vi "信号光谱7.vi"() -> ()   [LabVIEW 2018]
uses:
  <vilib>/Utility/NIReport.llb/Report Type.ctl
  <vilib>/Utility/file.llb/Write Delimited Spreadsheet (DBL).vi
  <vilib>/Instr/_visa.llb/VISA Configure Serial Port (Instr).vi
  <vilib>/addons/_office/excel.llb/Excel Get Data ([str]).vi
  <vilib>/Utility/NIReport.llb/NI_report.lvclass
  <vilib>/Analysis/NI_AALBase.lvlib
  <vilib>/ptbypt/NI_PtbyPt.lvlib
  <vilib>/Utility/NIReport.llb/NI_ReportGenerationCore.lvlib
  <vilib>/addons/_office/NI_ReportGenerationToolkit.lvlib
  <vilib>/Utility/NIReport.llb/Excel/NI_Excel.lvclass
panel:
  in  "终止测量":bool
  in  "测量次数":i32=10
  out "best fit":cluster{"Y":dbl[], "Y":dbl[]}[](graph)
  in  "拟合终点":i32=700
  in  "拟合起点":i32=350
  out "angle":dbl
  out "图片地址":string
  in  "开光时间/ms":u32=500
  out "最终存储路径 2":path
  out "照明光error out":errorcluster
  in  "照明光":bool
  in  "stop bits (10: 1 bit)":u16(ring)=10 items=["1.0"=10, "1.5"=15, "2.0"=20]
  in  "parity (0:none)":enum16{"None", "Odd", "Even", "Mark", "Space"}(ring)
  in  "data bits (8)":u16=8 min=5 max=8 step=1
  in  "baud rate":u32=9600 caption="baud rate (115200)" min=9600 max=115200
  in  "照明光VISA":refnum<visa-resource-name>="COM7"
  out "正在测量":bool
  in  "滤波阈值":dbl=1500.0 format="%#_13g"
  out "范围内？":bool[](array[boolean])
  out "w":dbl
  out "xc":dbl
  out "拟合参数":dbl[](array[numeric])
  out "最终存储路径":path
  in  "停止程序":bool
  in  "上升下降沿/s":dbl format="%.2p"
  in  "延时/s":dbl format="%.2p"
  in  "占空比/%":dbl=3.0 format="%.2p"
  in  "高电平/V":dbl=4.0 format="%.2p"
  in  "频率/Hz":dbl=6000.0 format="%.3p"
  in  "低电平/V":dbl min=0.0 max=5.0 format="%.2p"
  out "configure error out":errorcluster
  in  "设置参数":bool
  out "output control error  4":errorcluster
  in  "低电平持续输出":bool
  in  "Output 1":bool
  out "output control error  5":errorcluster
  in  "测量高电平/V":dbl=4.0
  out "output control error":errorcluster
  in  "开始测量":bool
  in  "上升下降沿":i32(ring)=1 items=["上升沿", "下降沿"]
  in  "channel输出口":i32(ring) items=["Channel 1", "Channel 2"]
  in  "输出信号波形":u16(ring) items=["Pulse"]
  out "output control error":errorcluster
  out "Output":bool
  in  "VISA 信号发生器":refnum<visa-resource-name>="USB0::0x1AB1::0x0641::DG4E192200870::INSTR"
  out "Spectrum":cluster{"Y":dbl[], "Y":dbl[]}[](graph)
  out "波长范围":dbl[](array[numeric])
  in  "选项卡控件":enum32{"IHR 550", "CCD"}(tab)
  in  "Move To\nTarget Positions":bool
  out "Current UniqueID":string="Mono4"
  in  "Mono ID":string(combo)="Mono1"
  in  "Connect":bool
  out "Initialized JY":bool=TRUE
  in  "Force\nInitialization":bool
  in  "Target Grating":string(combo)="2"
  out "Current Description":string="1" caption="Description"
  out "Grating Index":i32=1
  out "Current Grating":dbl=1200.0
  out "Units":string="nm"
  out "Current WL":dbl=897.9988
  out "Exit Mirror\nPosition":i32(ring)=2 items=["EntranceMirror", "ExitMirror", "Front", "Side"]
  out "Entrance Mirror\nPosition":i32(ring)=2 items=["EntranceMirror", "ExitMirror", "Front", "Side"]
  out "Units 2":string="mm"
  out "Front Entrance":dbl
  in  "Target WL":dbl=2670.0
  in  "Exit Mirror":u16(ring)=3 caption="Target Position Exit Mirror" items=["Front"=2, "Side"=3]
  in  "Entrance Mirror":u16(ring)=2 caption="Target Position\nEntrance Mirror" items=["Front"=2, "Side"=3]
  in  "Target\nFront Entrance":dbl=1.0
  in  "Commande tab":T1(tab)
  in  "Area Number to Display":i32
  in  "Reformat":bool
  in  "GAIN":u16(ring)=2 caption="Device Name" items=["High Light", "Best Dynamic Range", "High Sensitivity"]
  in  "ADC":u16(ring) caption="Device Name" items=["20 kHz       ", " 1 MHz       ", " 1 MHz Ultra "]
  in  "Number of Areas :":u16=1 min=1 step=1
  in  "Integration time (ms) :":i16=10000
  out "Uniques ID":u16(ring) items=["CCD1", "CCD2"]
  in  "Device Name":u16(ring) items=["Synapse CCD (Lateral)", "Synapse_IGA (Axial)"]
  in  "Signal type :":enum16{"TTL Rising Edge", "TTL Falling Edge"}(ring)=enum."TTL Falling Edge"
  in  "Trigger Type :":u16(ring) items=["On Start"=1, "Per Acquisition"=2]
  in  "trigSigTypeString":string
  in  "trigEventString":string
  in  "Enable InputTriggers :":bool
  in  "Number of Cleans":i32=1
  in  "MultiAcqShutterMode":i32(ring)=3 items=["Open For All Spectra"=1, "Open for Each Spectrum"=3]
  in  "Accumulations:":u16=10 min=1 step=1
  in  "Multi Accumulation mode:":bool
  out "Y Pixels:":i32=256
  out "DataSize":i32=1024
  out "X Pixels:":i32=1024
  out "Firmware\nVersion":string="V1.20 CCD_4000"
  out "initialized ?":bool=TRUE
  in  "Continuous":bool
  in  "CCD Busy":bool
  out "indicator":string="Ready !"
  in  "initialize":bool
  in  "ShutterOpen":bool=TRUE caption="Shutter enable"
  in  "Acquire":bool
  in  "Temperature":bool
  in  "Setup":bool
  out "Acq Time(ms)":u32=3401
  in  "Save Backlight":bool
  in  "cut backlight":bool
  out "backlight":bool=TRUE
  in  "是否拟合":bool
  in  "是否保存":bool
  in  "Close":bool=TRUE
  out "JYCCDLib.IJYCCDReqd":refnum<k7>
  out "areas :":i32[][](array[numeric])=[[1], [1], [1], [1024], [256], [1], [256]]
  in  "Constante de condition\n(Voir l'aide contextuelle)":bool
  out "temp graph":dbl(graph)=-134.538067
  out "ADC Number":i32[](array[numeric])=[0, 1, 2, 3, 4]
  out "Gain Number":i32[](array[numeric])=[10, 11, 12, 13, 8, 2]
  out "trigAddress":i32
  out "Data":i32[][](graph)
  out "error out":errorcluster
  out "Gratings":dbl[](array[numeric])=[1200.0, 300.0]
  out "Backlight":i32[][](graph)
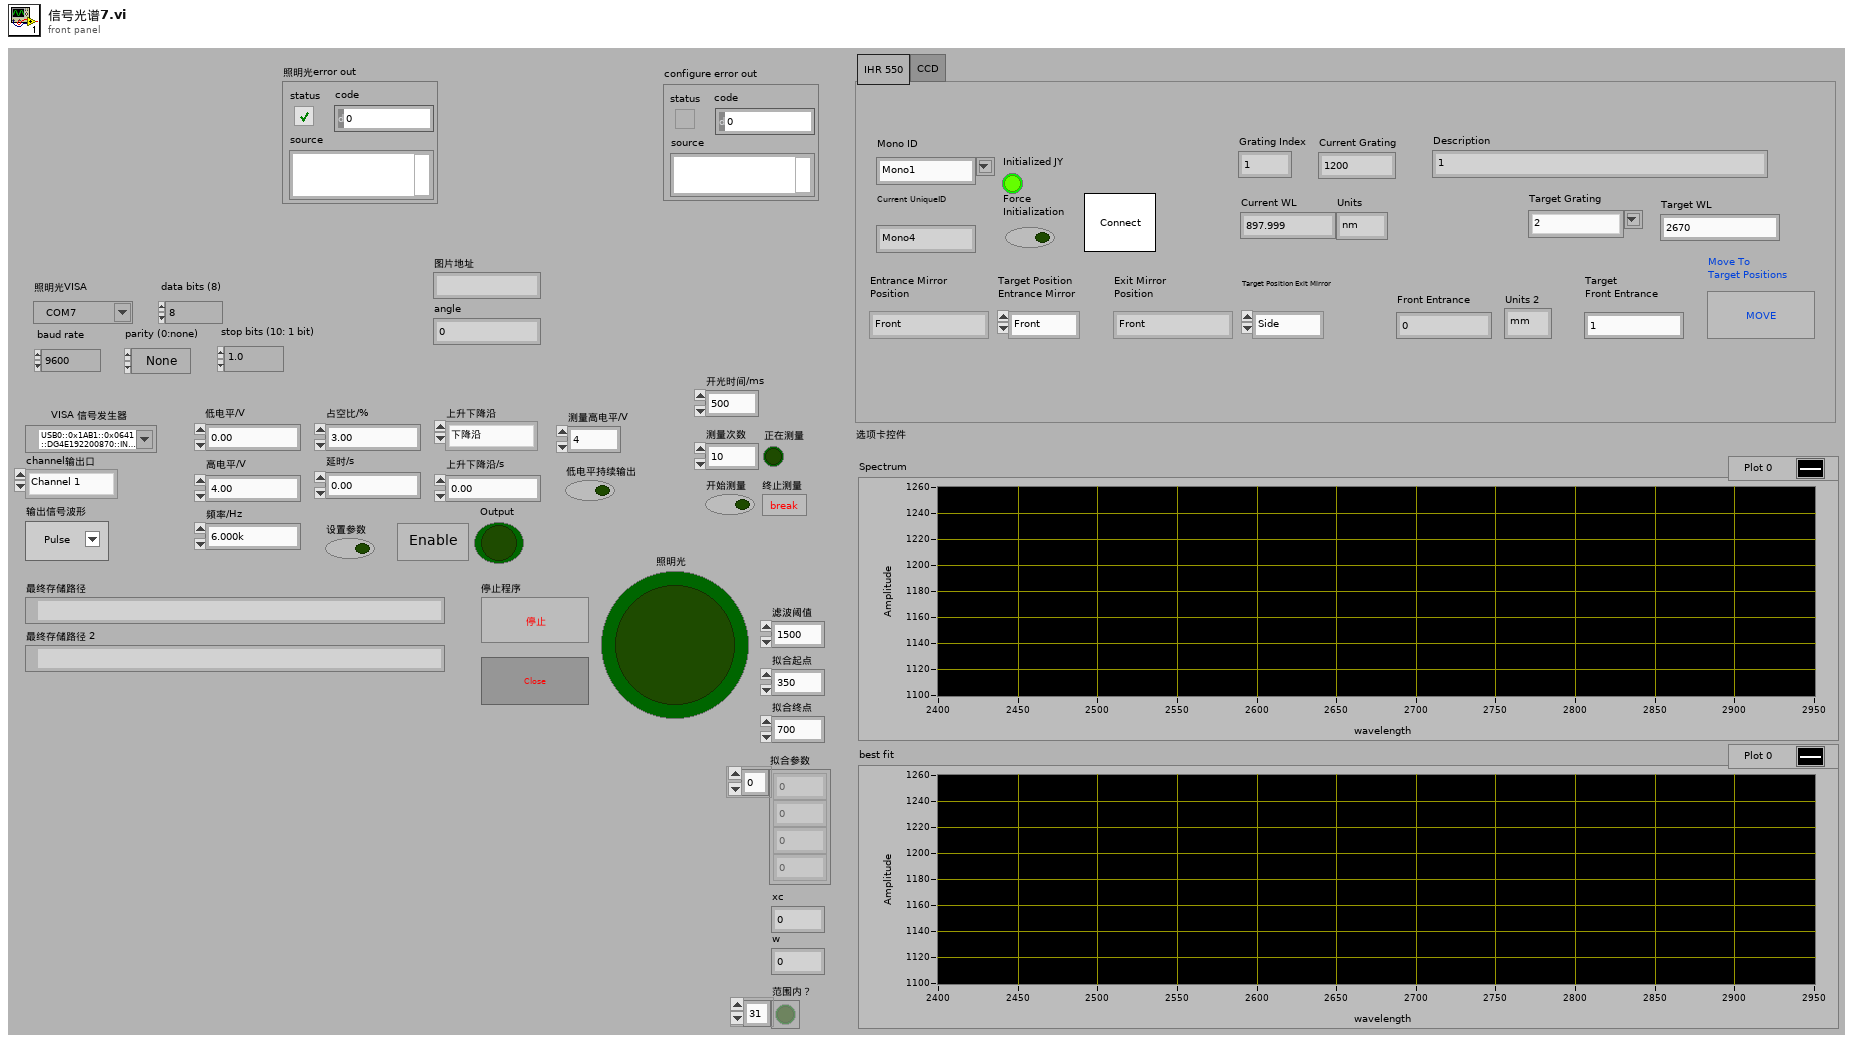
[diagram p1: front panel]
types:
  T1 = enum32{"Settings", "Trigger In", "Multi-Accu.", "Infos"}
  T2 = enum8{"Enabled", "Disabled", "Disabled and Grayed Out"}
  T3 = enum16{"maximized", "minimized", "normal", "no change"}
  T4 = typedef "NI_ReportGenerationCore.lvlib/Report Type.ctl" = enum16{"HTML", "Word", "Excel"}
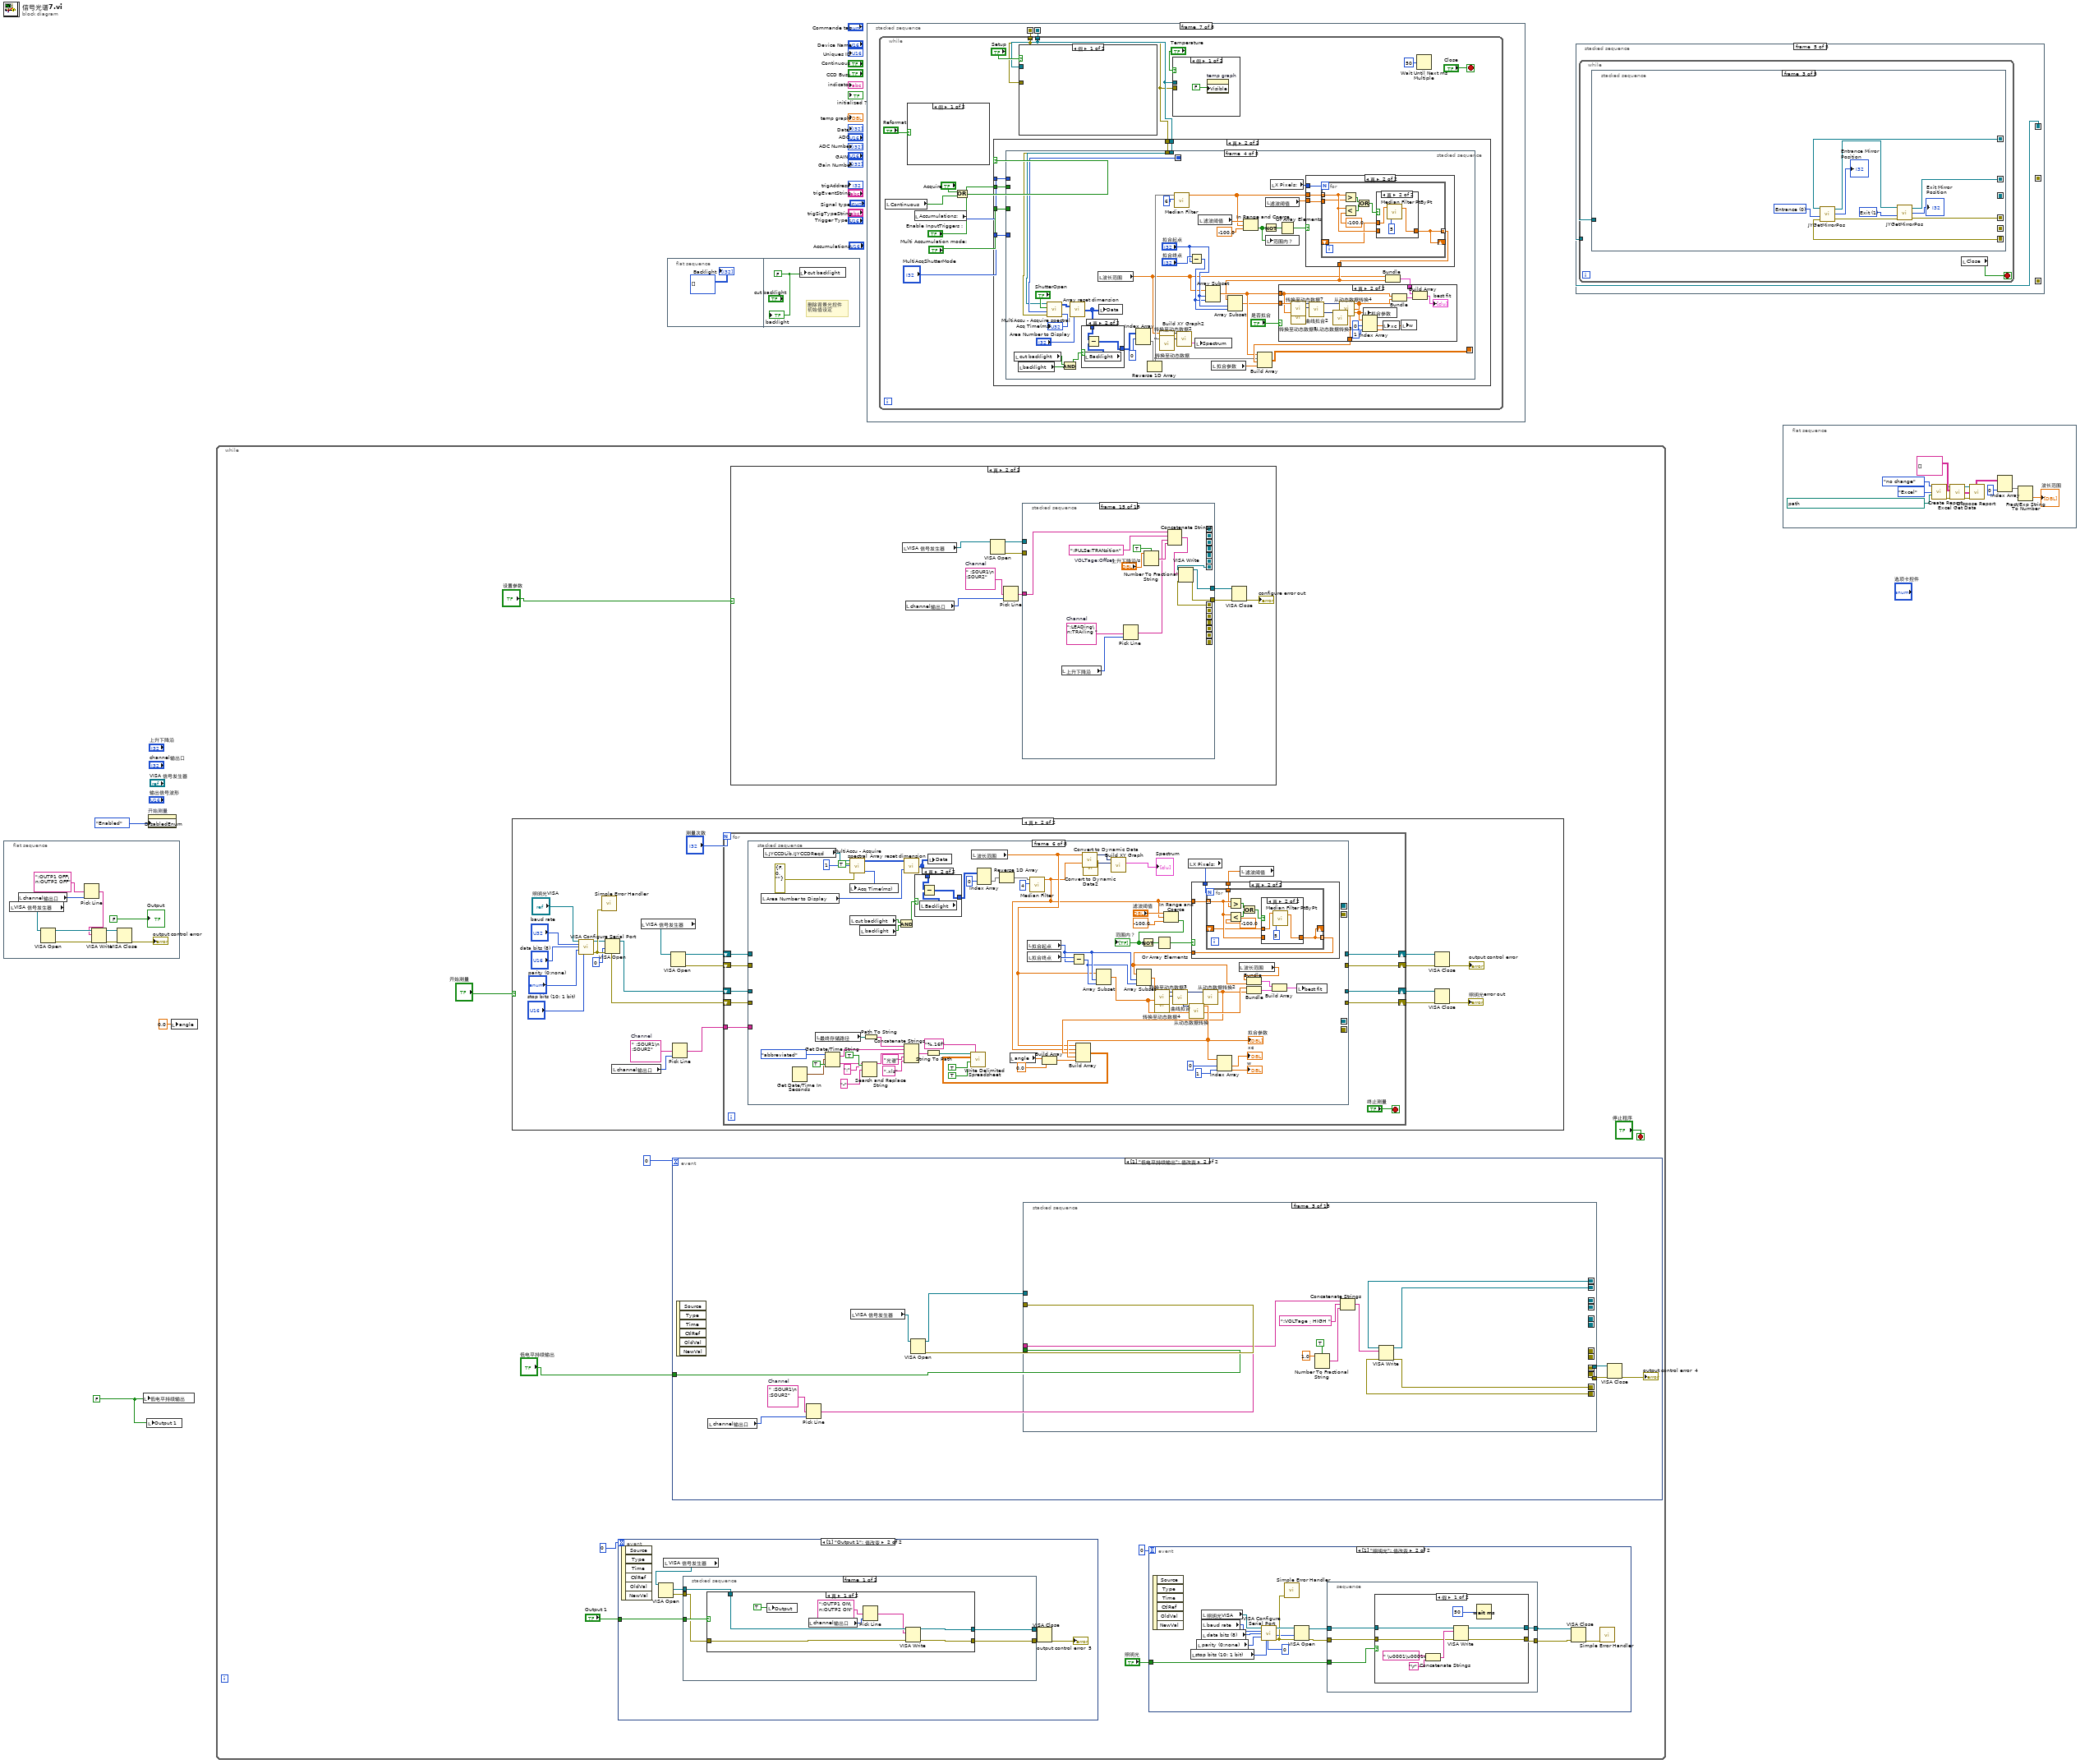
[diagram p0: block diagram]
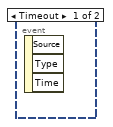
[diagram p2: hidden frame]
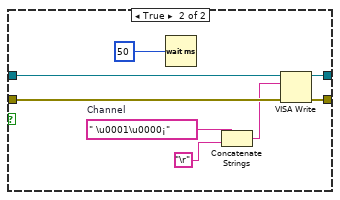
[diagram p3: hidden frame]
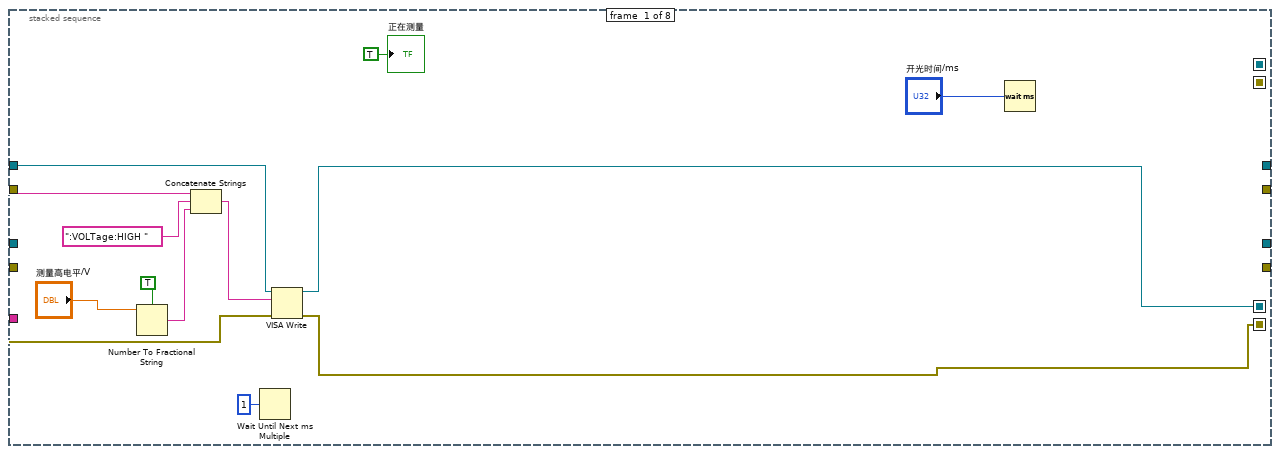
[diagram p5: hidden frame]
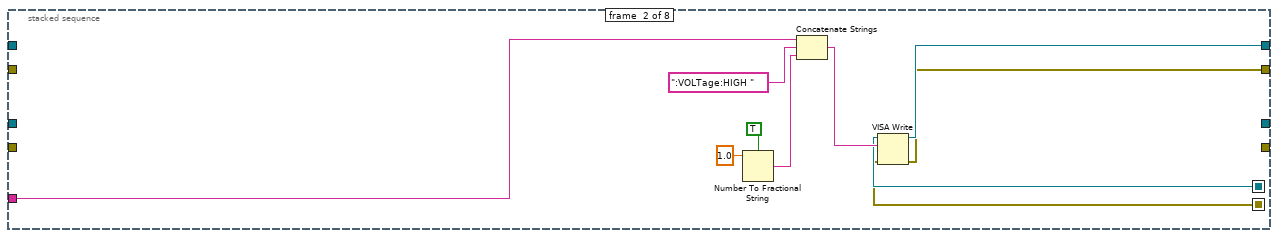
[diagram p6: hidden frame]
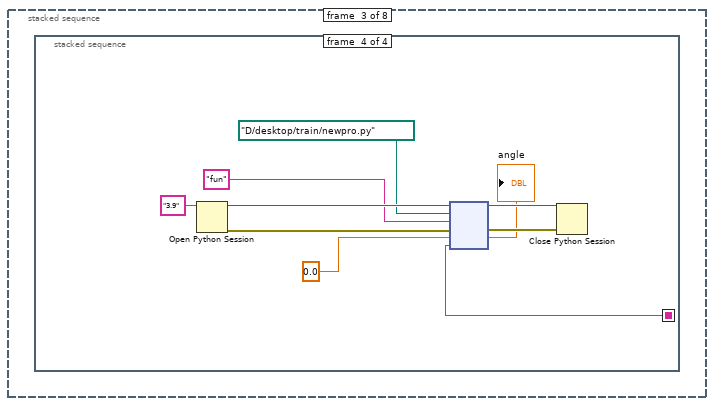
[diagram p7: hidden frame]
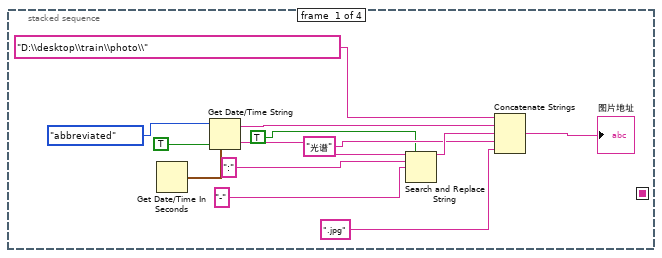
[diagram p8: hidden frame]
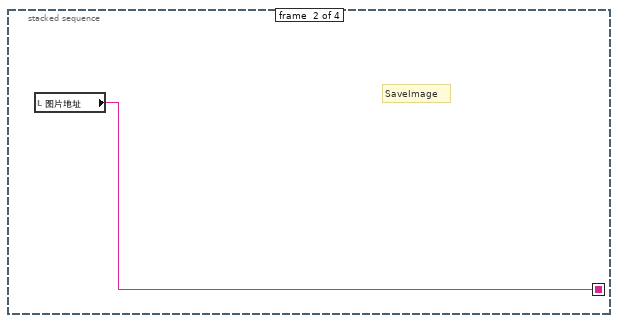
[diagram p9: hidden frame]
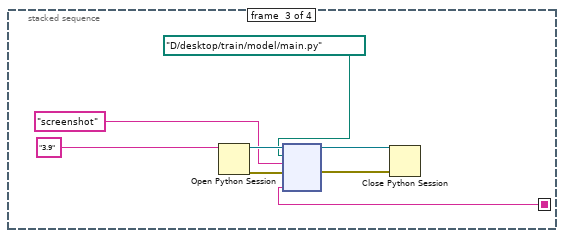
[diagram p10: hidden frame]
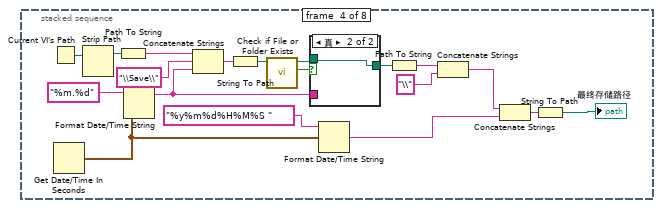
[diagram p11: hidden frame]
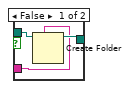
[diagram p12: hidden frame]
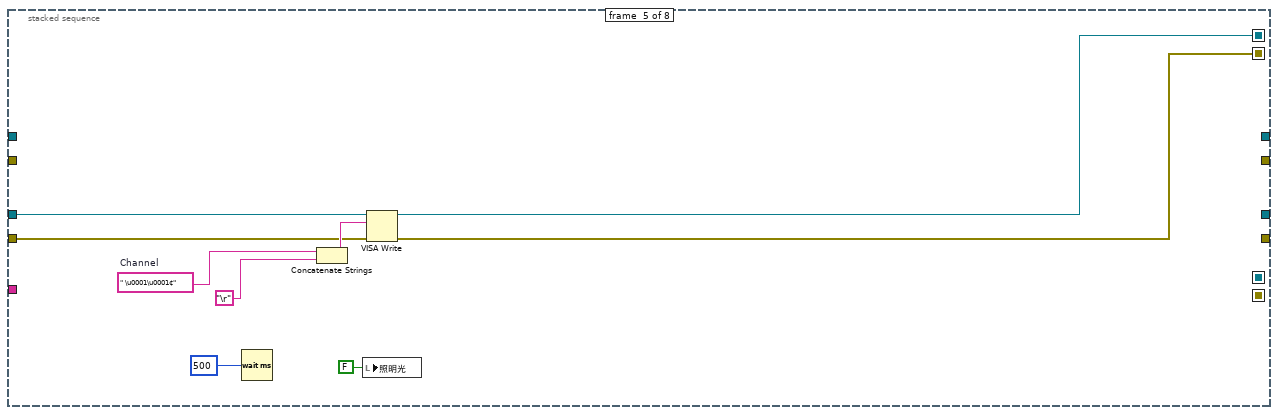
[diagram p13: hidden frame]
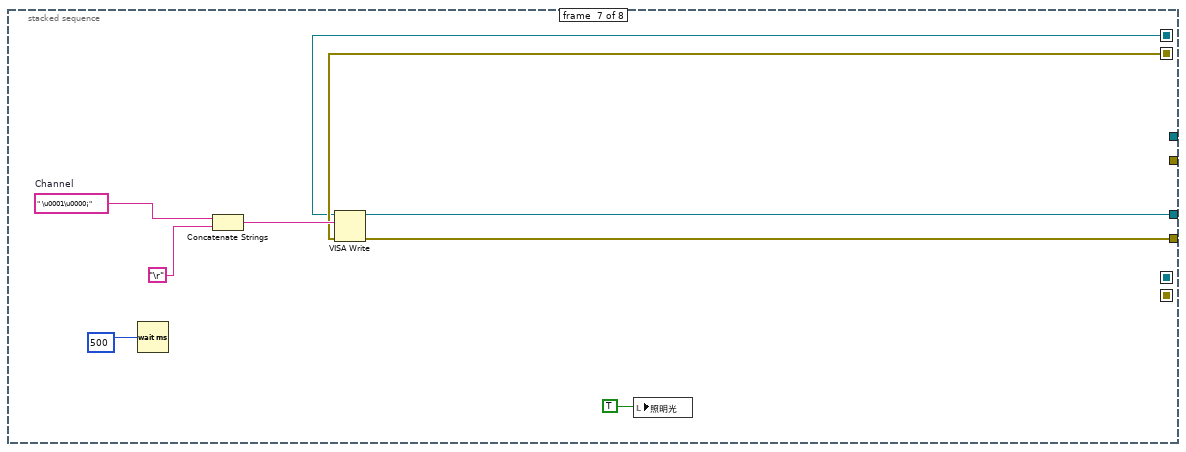
[diagram p17: hidden frame]
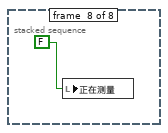
[diagram p18: hidden frame]
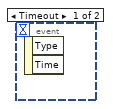
[diagram p19: hidden frame]
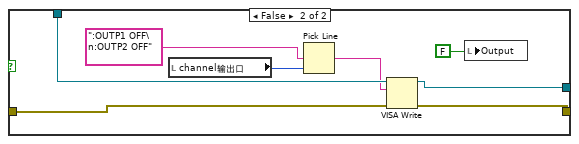
[diagram p20: hidden frame]
diagram:
  w2 = FALSE
  n1 = flat-sequence {
    frame #0 {
      n2 = local read "VISA 信号发生器"() -> (w7:refnum<visa-resource-name>)
      n3 = local read "channel输出口"() -> (w5:i32)
      n4 = VISA Open(VISA resource name=w7) -> (VISA resource name=w13:refnum<visa-resource-name>, error out=w12:errorcluster)  [unwired: 4 in]
      n5 = Pick Line(multi-line string=":OUTP1 OFF\n:OUTP2 OFF" ("write buffer"), line index=w5) -> (output string=w4:string)  [unwired: 1 in]
      n6 = VISA Write(VISA resource name=w13, write buffer=w4, error in (no error)=w12) -> (VISA resource name out=w10:refnum<visa-resource-name>, error out=w9:errorcluster)  [unwired: 1 out]
      n7 = VISA Close(VISA resource name=w10, error in (no error)=w9) -> (error out=→"output control error":errorcluster)
      "Output" <- FALSE ("布尔")
    }
  }
  n8 = local write "低电平持续输出"(w2) -> ()
  n9 = local write "Output 1"(w2) -> ()
  n10 = property on="开始测量" class="Bool"("DisabledEnum"=T2."Enabled" ("禁用")) -> ()  [unwired: 2 in, 2 out]
  n11 = local write "angle"(0.0 ("angle")) -> ()
  n12 = while {
    stop <- "停止程序" stop-if-true
    n13 = case shown="真" "开始测量" {
      frame False {
      }
      frame True {
        w74 = " :SOUR1\n :SOUR2"  # Channel
        n14 = call-poly "VISA Configure Serial Port"("VISA resource name"="照明光VISA", "baud rate (9600)"="baud rate", "data bits (8)"="data bits (8)", "parity (0:none)"="parity (0:none)", "stop bits (10: 1 bit)"="stop bits (10: 1 bit)") -> ("VISA resource name out"=w69:refnum<visa-resource-name>, "error out"=w70:errorcluster)  [unwired: 9 in]
        n15 = call <vilib>:"Simple Error Handler.vi"("error in (no error)"=w70) -> ()  [unwired: 4 in, 5 out]
        n16 = VISA Open(access mode=0, error in (no error)=w70, VISA resource name=w69) -> (VISA resource name=w62:refnum<visa-resource-name>, error out=w61:errorcluster)  [unwired: 2 in]
        n17 = local read "channel输出口"() -> (w75:i32)
        n18 = local read "VISA 信号发生器"() -> (w80:refnum<visa-resource-name>)
        n19 = VISA Open(VISA resource name=w80) -> (VISA resource name=w79:refnum<visa-resource-name>, error out=w78:errorcluster)  [unwired: 4 in]
        n20 = Pick Line(multi-line string=w74, line index=w75) -> (output string=w73:string)  [unwired: 1 in]
        n21 = for {
          N: "测量次数" -> [_]
          tunnel: w73 -> [w88]
          shift-right: [w84] -> w72
          shift-left: w79 -> [w90]
          shift-right: [w83] -> w71
          shift-left: w78 -> [w89]
          shift-right: [w82] -> w77
          shift-left: w62 -> [w87]
          shift-right: [w81] -> w76
          shift-left: w61 -> [w86]
          stop <- "终止测量" stop-if-true
          n22 = stacked-sequence {
            seq-local: [w95 _ _ _ _ _ _ _] -> [_ w106 _ _ _ _ _ _]
            seq-local: [w94 _ _ _ _ _ _ _] -> [_ w105 _ _ _ _ _ _]
            seq-local: [_ _ _ _ w171 _ _ _] -> [_ _ _ _ _ _ w271 _]
            seq-local: [_ _ _ _ w170 _ _ _] -> [_ _ _ _ _ _ w274 _]
            tunnel: w90 -> [w98 _ _ _ _ _ _ _]
            tunnel: w89 -> [w97 _ _ _ _ _ _ _]
            tunnel: [_ w108 _ _ _ _ _ _] -> w84
            tunnel: [_ w107 _ _ _ _ _ _] -> w83
            tunnel: w88 -> [w99 w104 _ _ _ _ _ _]
            tunnel: w87 -> [_ _ _ _ w174 _ _ _]
            tunnel: w86 -> [_ _ _ _ w173 _ _ _]
            tunnel: [_ _ _ _ _ _ w273 _] -> w82
            tunnel: [_ _ _ _ _ _ w272 _] -> w81
            frame #0 {
              n23 = Number To Fractional String(use system decimal point (T)=TRUE ("使用系统小数点(T)"), number="测量高电平/V") -> (F-format string=w101:string)  [unwired: 2 in]
              n24 = Concatenate Strings ("连接字符串")(w99, ":VOLTage:HIGH ", w101) -> (w100:string)
              n25 = Wait Until Next ms Multiple(millisecond multiple=u32 1 ("毫秒倍数")) -> ()  [unwired: 1 out]
              n26 = VISA Write(VISA resource name=w98, write buffer=w100, error in (no error)=w97) -> (VISA resource name out=w95:refnum<visa-resource-name>, error out=w94:errorcluster)  [unwired: 1 out]
              n27 = Wait (ms)(milliseconds to wait="开光时间/ms") -> ()  [unwired: 1 out]
              "正在测量" <- TRUE
            }
            frame #1 {
              n28 = Number To Fractional String(use system decimal point (T)=TRUE ("使用系统小数点(T)"), number=1.0 ("数字")) -> (F-format string=w111:string)  [unwired: 2 in]
              n29 = Concatenate Strings ("连接字符串")(w104, ":VOLTage:HIGH ", w111) -> (w110:string)
              n30 = VISA Write(VISA resource name=w106, write buffer=w110, error in (no error)=w105) -> (VISA resource name out=w108:refnum<visa-resource-name>, error out=w107:errorcluster)  [unwired: 1 out]
            }
            frame #2 {
              n31 = stacked-sequence {
                seq-local: [_ w127 _ _] -> [_ _ w128 w136]
                frame #0 {
                  n32 = Get Date/Time In Seconds() -> (seconds since 1Jan1904=w123:timestamp)
                  n33 = Get Date/Time String(date format (0)=enum16{"short", "long", "abbreviated"}."abbreviated" ("日期格式(0)"), seconds (now)=w123, want seconds? (F)=TRUE ("需要秒？(F)")) -> (date string=w126:string, time string=w124:string)
                  n34 = Search and Replace String(replace all?=TRUE ("替换全部？(F)"), input string=w124, search string=":" ("搜索字符串"), replace string="-" ("替换字符串(\"\")")) -> (result string=w125:string)  [unwired: 4 in, 3 out]
                  n35 = Concatenate Strings("D:\\desktop\\train\\photo\\", w126, w125, "光谱" ("字符串"), ".jpg" ("字符串")) -> (→"图片地址":string)
                }
                frame #1 {
                  # "SaveImage"
                  n36 = local read "图片地址"() -> (w127:string)
                }
                frame #2 {
                  n37 = Open Python Session(python version="3.9" ("Python version")) -> (session out=w135:refnum<k35>, error out=w133:errorcluster)  [unwired: 2 in]
                  n38 = node(w135, path "D:/desktop/train/model/main.py" ("module path"), "screenshot" ("function name"), w133, w128) -> (w134:refnum<k35>, w132:errorcluster)  [unwired: 3 in, 2 out]
                  n39 = Close Python Session(session in=w134, error in=w132) -> ()  [unwired: 1 out]
                }
                frame #3 {
                  n40 = Open Python Session(python version="3.9" ("Python version")) -> (session out=w144:refnum<k35>, error out=w142:errorcluster)  [unwired: 2 in]
                  n41 = node(w144, path "D:/desktop/train/newpro.py" ("module path"), "fun" ("function name"), w142, 0.0, w136) -> (w143:refnum<k35>, w141:errorcluster, →"angle":dbl)  [unwired: 1 in, 2 out]
                  n42 = Close Python Session(session in=w143, error in=w141) -> ()  [unwired: 1 out]
                }
              }
            }
            frame #3 {
              n43 = Current VI's Path() -> (path=w151:path)
              n44 = Get Date/Time In Seconds() -> (seconds since 1Jan1904=w153:timestamp)
              n45 = Strip Path(path=w151) -> (stripped path=w152:path)  [unwired: 1 out]
              n46 = Path To String(path=w152) -> (string=w154:string)
              n47 = Format Date/Time String(time format string (%c)="%m.%d" ("时间格式字符串(%c)"), seconds (now)=w153) -> (date/time string=w160:string)  [unwired: 1 in]
              n48 = Concatenate Strings(w154, "\\Save\\" ("字符串"), w160) -> (w155:string)
              n49 = String To Path(string=w155) -> (path=w156:path)
              n50 = call <vilib>:"Check if File or Folder Exists.vi"("path"=w156) -> ("file or folder exists?"=w157:bool, "dup path"=w159:path)  [unwired: 8 in, 1 out]
              n51 = case shown="真" w157 {
                tunnel: [w167 w168] -> w158
                tunnel: w159 -> [w166 w168]
                tunnel: w160 -> [w165 _]
                frame False {
                  n52 = Create Folder(prompt (Create Folder)=w165, path (use dialog)=w166) -> (created path=w167:path)  [unwired: 1 in, 2 out]
                }
                frame True {
                }
              }
              n53 = Format Date/Time String(time format string (%c)="%y%m%d%H%M%S " ("时间格式字符串(%c)"), seconds (now)=w153) -> (date/time string=w163:string)  [unwired: 1 in]
              n54 = Path To String(path=w158) -> (string=w161:string)
              n55 = Concatenate Strings(w161, "\\" ("字符串")) -> (w162:string)
              n56 = Concatenate Strings(w162, w163) -> (w150:string)
              n57 = String To Path(string=w150) -> (path=→"最终存储路径":path)
            }
            frame #4 {
              w169 = " \u0001\u0001¢"  # Channel
              n58 = Wait (ms)(milliseconds to wait=500) -> ()  [unwired: 1 out]
              n59 = Concatenate Strings(w169, "\r") -> (w175:string)
              n60 = local write "照明光"(FALSE ("照明光")) -> ()
              n61 = VISA Write(VISA resource name=w174, write buffer=w175, error in (no error)=w173) -> (VISA resource name out=w171:refnum<visa-resource-name>, error out=w170:errorcluster)  [unwired: 1 out]
            }
            frame #5 {
              n62 = local read "Area Number to Display"() -> (w221:i32)
              n63 = local read "JYCCDLib.IJYCCDReqd"() -> (w217:refnum<k7>)
              n64 = Get Date/Time In Seconds() -> (seconds since 1Jan1904=w230:timestamp)
              n65 = local read "最终存储路径"() -> (w244:path)
              n66 = Get Date/Time String(date format (0)=enum16{"short", "long", "abbreviated"}."abbreviated" ("日期格式(0)"), seconds (now)=w230, want seconds? (F)=TRUE ("需要秒？(F)")) -> (date string=w238:string, time string=w233:string)
              n67 = call "MultiAccu - Acquire spectral.vi"("error in"=errorcluster {"status"=FALSE, "code"=0, "source"=""}, "Accumulations:"=u16 1, "ShutterOpen"=TRUE, "JYCCDLib.IJYCCDReqd"=w217) -> ("Acq Time(ms)"=w223:u32, "Array Out"=w222:i32[][][])  [unwired: 1 out]
              n68 = local write "Acq Time(ms)"(w223) -> ()
              n69 = local read "cut backlight"() -> (w203:bool)
              n70 = local read "backlight"() -> (w201:bool)
              n71 = Search and Replace String(replace all?=TRUE ("替换全部？(F)"), input string=w233, search string=":" ("搜索字符串"), replace string="-" ("替换字符串(\"\")")) -> (result string=w237:string)  [unwired: 4 in, 3 out]
              n72 = Path To String(path=w244) -> (string=w227:string)
              n73 = And(x=w203, y=w201) -> (x .and. y?=w202:bool)
              n74 = call "Array reset dimension.vi"("Area Number"=w221, "Array In"=w222) -> ("Array Out"=w205:i32[][])
              n75 = Concatenate Strings(w227, w238, w237, "光谱" ("字符串"), ".xls" ("字符串")) -> (w242:string)
              n76 = case shown="真" w202 {
                tunnel: [w265 w267] -> w204
                tunnel: w205 -> [w265 w266]
                frame False {
                }
                frame True {
                  n77 = local read "Backlight"() -> (w268:i32[][])
                  n78 = Subtract(x=w266, y=w268) -> (x-y=w267:i32[][])
                }
              }
              n79 = String To Path(string=w242) -> (path=w243:path)
              n80 = local write "Data"(w205) -> ()
              n81 = local read "波长范围"() -> (w182:dbl[])
              n82 = Index Array(array=w204, index (row)=0 ("索引 (行)")) -> (element=w245:i32[])  [unwired: 1 in]
              n83 = Reverse 1D Array(array=w245) -> (reversed array=w246:i32[])
              n84 = local read "angle"() -> (w180:dbl)
              n85 = local read "拟合起点"() -> (w191:i32)
              n86 = local read "拟合终点"() -> (w193:i32)
              n87 = call <vilib>:"Median Filter.vi"("left rank"=4, "X"=w246) -> ("Filtered X"=w181:dbl[])  [unwired: 8 in, 1 out]
              n88 = Build Array(w180, 0.0 ("元素")) -> (w178:dbl[])
              n89 = Subtract(x=w193, y=w191) -> (x-y=w190:i32)
              n90 = call "Convert to Dynamic Data"("Array"=w182) -> ("Dynamic Data Type"=w214:dynamicdata)  [unwired: 3 in]
              n91 = call "Convert to Dynamic Data2"("Array"=w181) -> ("Dynamic Data Type"=w213:dynamicdata)  [unwired: 3 in]
              n92 = Array Subset(array=w182, index=w191, length=w190) -> (w188:dbl[])
              n93 = call "Build XY Graph"("Y Input"=w213, "X Input"=w214) -> ("XY Graph"=→"Spectrum":cluster{"Y":dbl[], "Y":dbl[]}[])  [unwired: 8 in, 1 out]
              n94 = call "转换至动态数据4"("Array"=w188) -> ("Dynamic Data Type"=w211:dynamicdata)  [unwired: 3 in]
              n95 = In Range and Coerce(upper limit="滤波阈值", x=w181, lower limit=-100.0) -> (In Range?=w196:bool[])  [unwired: 1 out]
              "范围内？" <- w196
              n96 = Not(x=w196) -> (.not. x?=w195:bool[])
              n97 = Or Array Elements(Boolean array=w195) -> (logical OR=w198:bool)
              n98 = local read "X Pixels:"() -> (w197:i32)
              n99 = local read "波长范围"() -> (w183:dbl[])
              n100 = local read "滤波阈值"() -> (w194:dbl)
              n101 = case shown="真" w198 {
                tunnel: w197 -> [_ w252]
                tunnel: w181 -> [w248 w251]
                tunnel: [w248 w250] -> w189
                tunnel: w194 -> [_ w249]
                frame False {
                }
                frame True {
                  n102 = for {
                    N: w252 -> [_]
                    tunnel: w251 -> [w256] mode=indexing
                    tunnel: [w255] -> w250 mode=indexing
                    shift-right: [w255] -> _
                    shift-left: _ -> [w254]
                    tunnel: w249 -> [w253]
                    n103 = Greater?(x=w256, y=w253) -> (0:w258:bool)
                    n104 = Less?(x=w256, y=-100.0) -> (x < y?=w259:bool)
                    n105 = Or(x=w258, y=w259) -> (x .or. y?=w257:bool)
                    n106 = case shown="真" w257 {
                      tunnel: w256 -> [w261 _]
                      tunnel: [w261 w263] -> w255
                      tunnel: w254 -> [_ w264]
                      frame False {
                      }
                      frame True {
                        n107 = call <vilib>:"Median Filter PtByPt.vi"("rank"=5, "x"=w264) -> ("Filtered x"=w263:dbl)  [unwired: 2 in, 1 out]
                      }
                    }
                  }
                }
              }
              n108 = Array Subset(array=w189, index=w191, length=w190) -> (w192:dbl[])
              n109 = call "转换至动态数据3"("Array"=w192) -> ("Dynamic Data Type"=w212:dynamicdata)  [unwired: 3 in]
              n110 = call "曲线拟合"("Locations"=w211, "Signals"=w212) -> ("best fit"=w216:dynamicdata, "non-linear coefficients"=w215:dynamicdata)  [unwired: 5 in, 3 out]
              n111 = call "从动态数据转换"("Dynamic Data Type"=w215) -> ("Array"=w208:dbl[])  [unwired: 3 in]
              "拟合参数" <- w208
              n112 = call "从动态数据转换2"("Dynamic Data Type"=w216) -> ("Array"=w187:dbl[])  [unwired: 3 in]
              n113 = Build Array(w182, w181, w187, w208, w178) -> (w247:dbl[][])
              n114 = call-poly <vilib>:"Write Delimited Spreadsheet.vi"("file path (dialog if empty)"=w243, "format (%.3f)"="%.16f", "2D data"=w247, "append to file? (new file:F)"=TRUE ("append to file? (F)"), "transpose? (no:F)"=TRUE ("transpose? (F)")) -> ()  [unwired: 9 in, 2 out]
              n115 = Index Array(array=w208, index #1=0 ("索引"), index #2=1 ("索引")) -> (element #1=→"xc":dbl, element #2=→"w":dbl)
              n116 = Bundle("波长范围"=w183, "Filtered X"=w189) -> (w186:cluster{"波长范围 ":dbl[], "Filtered X":dbl[]})  [unwired: 1 in]
              n117 = Bundle(w188, "Array"=w187) -> (w185:cluster{dbl[], "Array":dbl[]})  [unwired: 1 in]
              n118 = Build Array(w186, w185) -> (w184:cluster{"波长范围 ":dbl[], "Array":dbl[]}[])
              n119 = local write "best fit"(w184) -> ()
            }
            frame #6 {
              w269 = " \u0001\u0000¡"  # Channel
              n120 = Wait (ms)(milliseconds to wait=500) -> ()  [unwired: 1 out]
              n121 = Concatenate Strings(w269, "\r") -> (w275:string)
              n122 = VISA Write(VISA resource name=w271, write buffer=w275, error in (no error)=w274) -> (VISA resource name out=w273:refnum<visa-resource-name>, error out=w272:errorcluster)  [unwired: 1 out]
              n123 = local write "照明光"(TRUE ("照明光")) -> ()
            }
            frame #7 {
              n124 = local write "正在测量"(FALSE) -> ()
            }
          }
        }
        n125 = VISA Close(VISA resource name=w72, error in (no error)=w71) -> (error out=→"output control error":errorcluster)
        n126 = VISA Close(VISA resource name=w77, error in (no error)=w76) -> (error out=→"照明光error out":errorcluster)
      }
    }
    n127 = event shown="[1] \"Output 1\": 值改变" {
      selector: _ -> [_ _]
      dyn-events: _ -> [_ _]
      timeout: u32 0 ("Time") -> [_ _]
      tunnel: "Output 1" -> [_ w283]
      event Timeout {
        n128 = event-data() -> ()  [unwired: 1 in, 2 out]
      }
      event "Output 1": Value Change {
        n129 = event-data() -> ()  [unwired: 1 in, 6 out]
        n130 = local read "VISA 信号发生器"() -> (w279:refnum<visa-resource-name>)
        n131 = VISA Open(VISA resource name=w279) -> (VISA resource name=w282:refnum<visa-resource-name>, error out=w285:errorcluster)  [unwired: 4 in]
        n132 = stacked-sequence {
          tunnel: w283 -> [w290 _]
          tunnel: w285 -> [w289 _]
          tunnel: w282 -> [w288 _]
          tunnel: [w287 _] -> w281
          tunnel: [w286 _] -> w280
          frame #0 {
            n133 = case shown="真" w290 {
              tunnel: w288 -> [w298 w306]
              tunnel: [w297 w305] -> w286
              tunnel: w289 -> [w296 w303]
              tunnel: [w295 w304] -> w287
              frame True {
                n134 = local write "Output"(TRUE ("布尔")) -> ()
                n135 = local read "channel输出口"() -> (w292:i32)
                n136 = Pick Line(multi-line string=":OUTP1 ON\n:OUTP2 ON" ("write buffer"), line index=w292) -> (output string=w291:string)  [unwired: 1 in]
                n137 = VISA Write(VISA resource name=w298, write buffer=w291, error in (no error)=w296) -> (VISA resource name out=w295:refnum<visa-resource-name>, error out=w297:errorcluster)  [unwired: 1 out]
              }
              frame False {
                n138 = local read "channel输出口"() -> (w300:i32)
                n139 = Pick Line(multi-line string=":OUTP1 OFF\n:OUTP2 OFF" ("write buffer"), line index=w300) -> (output string=w299:string)  [unwired: 1 in]
                n140 = VISA Write(VISA resource name=w306, write buffer=w299, error in (no error)=w303) -> (VISA resource name out=w304:refnum<visa-resource-name>, error out=w305:errorcluster)  [unwired: 1 out]
                n141 = local write "Output"(FALSE ("布尔")) -> ()
              }
            }
          }
          frame #1 {
            n142 = Wait (ms)(milliseconds to wait=u32 150) -> ()  [unwired: 1 out]
          }
        }
        n143 = VISA Close(VISA resource name=w281, error in (no error)=w280) -> (error out=→"output control error  5":errorcluster)
      }
    }
    n144 = event shown="[1] \"低电平持续输出\": 值改变" {
      selector: _ -> [_ _]
      dyn-events: _ -> [_ _]
      timeout: u32 0 ("Time") -> [_ _]
      tunnel: "低电平持续输出" -> [_ w308]
      event Timeout {
        n145 = event-data() -> ()  [unwired: 1 in, 2 out]
      }
      event "低电平持续输出": Value Change {
        w312 = " :SOUR1\n :SOUR2"  # Channel
        n146 = event-data() -> ()  [unwired: 1 in, 6 out]
        n147 = local read "channel输出口"() -> (w313:i32)
        n148 = Pick Line(multi-line string=w312, line index=w313) -> (output string=w311:string)  [unwired: 1 in]
        n149 = local read "VISA 信号发生器"() -> (w316:refnum<visa-resource-name>)
        n150 = VISA Open(VISA resource name=w316) -> (VISA resource name=w315:refnum<visa-resource-name>, error out=w314:errorcluster)  [unwired: 4 in]
        n151 = stacked-sequence {
          seq-local: [w322 _ _ _ _ _ _ _ _ _ _ _ _] -> [_ _ w337 _ _ _ _ _ _ _ _ _ _]
          seq-local: [w321 _ _ _ _ _ _ _ _ _ _ _ _] -> [_ _ w336 _ _ _ _ _ _ _ _ _ _]
          seq-local: [_ _ w335 _ _ _ _ _ _ _ _ _ _] -> [_ _ _ _ w340 _ _ _ _ _ _ _ _]
          seq-local: [_ _ w334 _ _ _ _ _ _ _ _ _ _] -> [_ _ _ _ w341 _ _ _ _ _ _ _ _]
          seq-local: [_ _ _ _ w349 _ _ _ _ _ _ _ _] -> [_ _ _ _ _ _ w360 _ _ _ _ _ _]
          seq-local: [_ _ _ _ w348 _ _ _ _ _ _ _ _] -> [_ _ _ _ _ _ w359 _ _ _ _ _ _]
          seq-local: [_ _ _ _ _ _ w353 _ _ _ _ _ _] -> [_ _ _ _ _ _ _ _ w363 _ _ _ _]
          seq-local: [_ _ _ _ _ _ w352 _ _ _ _ _ _] -> [_ _ _ _ _ _ _ _ w362 _ _ _ _]
          seq-local: [_ _ _ _ _ _ _ _ w366 _ _ _ _] -> [_ _ _ _ _ _ _ _ _ _ w377 _ _]
          seq-local: [_ _ _ _ _ _ _ _ w365 _ _ _ _] -> [_ _ _ _ _ _ _ _ _ _ w376 _ _]
          seq-local: [_ _ _ _ _ _ _ _ _ _ w374 _ _] -> [_ _ _ _ _ _ _ _ _ _ _ _ w391]
          seq-local: [_ _ _ _ _ _ _ _ _ _ w373 _ _] -> [_ _ _ _ _ _ _ _ _ _ _ _ w390]
          tunnel: w315 -> [w327 _ _ _ _ _ _ _ _ _ _ _ _]
          tunnel: w314 -> [w320 _ _ _ _ _ _ _ _ _ _ _ _]
          tunnel: w311 -> [w319 _ w333 _ w346 _ w357 _ w367 _ w380 _ _]
          tunnel: [_ _ _ _ _ _ _ _ _ _ _ _ w389] -> w310
          tunnel: [_ _ _ _ _ _ _ _ _ _ _ _ w387] -> w309
          tunnel: w308 -> [_ _ _ _ _ _ _ _ _ _ _ _ w388]
          frame #0 {
            w324 = " PULSe"  # Function Command
            n152 = local read "输出信号波形"() -> (w318:u16)
            n153 = Concatenate Strings(w319, ":FUNC" ("string (\"\")")) -> (w325:string)
            n154 = Pick Line(string ("")=w325, multi-line string=w324, line index=w318) -> (output string=w323:string)
            n155 = VISA Write(VISA resource name=w327, write buffer=w323, error in (no error)=w320) -> (VISA resource name out=w322:refnum<visa-resource-name>, error out=w321:errorcluster)  [unwired: 1 out]
          }
          frame #1 {
            n156 = Wait (ms)(milliseconds to wait=u32 150) -> ()  [unwired: 1 out]
          }
          frame #2 {
            n157 = Number To Fractional String(use system decimal point (T)=TRUE ("使用系统小数点(T)"), number=1.0 ("数字")) -> (F-format string=w331:string)  [unwired: 2 in]
            n158 = Concatenate Strings ("连接字符串")(w333, ":VOLTage：HIGH ", w331) -> (w330:string)
            n159 = VISA Write(VISA resource name=w337, write buffer=w330, error in (no error)=w336) -> (VISA resource name out=w335:refnum<visa-resource-name>, error out=w334:errorcluster)  [unwired: 1 out]
          }
          frame #3 {
            n160 = Wait (ms)(milliseconds to wait=u32 150) -> ()  [unwired: 1 out]
          }
          frame #4 {
            # "1 电压偏置"
            n161 = Number To Fractional String(use system decimal point (T)=TRUE ("使用系统小数点(T)"), number=0.0 ("数字")) -> (F-format string=w344:string)  [unwired: 2 in]
            n162 = Concatenate Strings(w346, ":VOLTage:LOW ", w344) -> (w345:string)
            n163 = VISA Write(VISA resource name=w340, write buffer=w345, error in (no error)=w341) -> (VISA resource name out=w349:refnum<visa-resource-name>, error out=w348:errorcluster)  [unwired: 1 out]
          }
          frame #5 {
            n164 = Wait (ms)(milliseconds to wait=u32 150) -> ()  [unwired: 1 out]
          }
          frame #6 {
            n165 = local read "channel输出口"() -> (w355:i32)
            n166 = Pick Line(multi-line string=":OUTP1:IMPedance \n:OUTP2:IMPedance " ("write buffer"), line index=w355) -> (output string=w354:string)  [unwired: 1 in]
            n167 = Concatenate Strings ("连接字符串")(w357, w354, "INFINITY") -> (w358:string)
            n168 = VISA Write(VISA resource name=w360, write buffer=w358, error in (no error)=w359) -> (VISA resource name out=w353:refnum<visa-resource-name>, error out=w352:errorcluster)  [unwired: 1 out]
          }
          frame #7 {
            n169 = Wait (ms)(milliseconds to wait=u32 150) -> ()  [unwired: 1 out]
          }
          frame #8 {
            n170 = Number To Fractional String(use system decimal point (T)=TRUE ("使用系统小数点(T)"), number=0.0 ("数字")) -> (F-format string=w370:string)  [unwired: 2 in]
            n171 = Concatenate Strings(w367, ":PULSe:DELay ", w370) -> (w368:string)
            n172 = VISA Write(VISA resource name=w363, write buffer=w368, error in (no error)=w362) -> (VISA resource name out=w366:refnum<visa-resource-name>, error out=w365:errorcluster)  [unwired: 1 out]
          }
          frame #9 {
            n173 = Wait (ms)(milliseconds to wait=u32 150) -> ()  [unwired: 1 out]
          }
          frame #10 {
            w381 = ":LEADing\n:TRAiling "  # Channel
            w385 = ":PULSe:TRANsition"  # VOLTage:Offset
            n174 = local read "上升下降沿"() -> (w382:i32)
            n175 = Pick Line(multi-line string=w381, line index=w382) -> (output string=w378:string)  [unwired: 1 in]
            n176 = Number To Fractional String(use system decimal point (T)=TRUE ("使用系统小数点(T)"), number=0.0 ("数字")) -> (F-format string=w379:string)  [unwired: 2 in]
            n177 = Concatenate Strings(w380, w385, w378, w379) -> (w383:string)
            n178 = VISA Write(VISA resource name=w377, write buffer=w383, error in (no error)=w376) -> (VISA resource name out=w374:refnum<visa-resource-name>, error out=w373:errorcluster)  [unwired: 1 out]
          }
          frame #11 {
            n179 = Wait (ms)(milliseconds to wait=u32 150) -> ()  [unwired: 1 out]
          }
          frame #12 {
            n180 = case shown="假" w388 {
              tunnel: w391 -> [w399 w400]
              tunnel: [w398 w407] -> w387
              tunnel: w390 -> [w397 w405]
              tunnel: [w396 w406] -> w389
              frame True {
                n181 = local write "Output"(TRUE ("布尔")) -> ()
                n182 = local read "channel输出口"() -> (w393:i32)
                n183 = Pick Line(multi-line string=":OUTP1 ON\n:OUTP2 ON" ("write buffer"), line index=w393) -> (output string=w392:string)  [unwired: 1 in]
                n184 = VISA Write(VISA resource name=w399, write buffer=w392, error in (no error)=w397) -> (VISA resource name out=w396:refnum<visa-resource-name>, error out=w398:errorcluster)  [unwired: 1 out]
              }
              frame False {
                n185 = local read "channel输出口"() -> (w402:i32)
                n186 = Pick Line(multi-line string=":OUTP1 OFF\n:OUTP2 OFF" ("write buffer"), line index=w402) -> (output string=w401:string)  [unwired: 1 in]
                n187 = VISA Write(VISA resource name=w400, write buffer=w401, error in (no error)=w405) -> (VISA resource name out=w406:refnum<visa-resource-name>, error out=w407:errorcluster)  [unwired: 1 out]
                n188 = local write "Output"(FALSE ("布尔")) -> ()
              }
            }
          }
        }
        n189 = VISA Close(VISA resource name=w310, error in (no error)=w309) -> (error out=→"output control error  4":errorcluster)
      }
    }
    n190 = case shown="真" "设置参数" {
      frame False {
      }
      frame True {
        w413 = " :SOUR1\n :SOUR2"  # Channel
        n191 = local read "VISA 信号发生器"() -> (w409:refnum<visa-resource-name>)
        n192 = local read "channel输出口"() -> (w408:i32)
        n193 = VISA Open(VISA resource name=w409) -> (VISA resource name=w415:refnum<visa-resource-name>, error out=w416:errorcluster)  [unwired: 4 in]
        n194 = Pick Line(multi-line string=w413, line index=w408) -> (output string=w412:string)  [unwired: 1 in]
        n195 = stacked-sequence {
          seq-local: [w421 _ _ _ _ _ _ _ _ _ _ _ _ _ _] -> [_ _ w436 _ _ _ _ _ _ _ _ _ _ _ _]
          seq-local: [w420 _ _ _ _ _ _ _ _ _ _ _ _ _ _] -> [_ _ w435 _ _ _ _ _ _ _ w474 _ _ _ _]
          seq-local: [_ _ w434 _ _ _ _ _ _ _ _ _ _ _ _] -> [_ _ _ _ w445 _ _ _ _ _ _ _ _ _ _]
          seq-local: [_ _ w433 _ _ _ _ _ _ _ _ _ _ _ _] -> [_ _ _ _ w444 _ _ _ _ _ _ _ _ _ _]
          seq-local: [_ _ _ _ w443 _ _ _ _ _ _ _ _ _ _] -> [_ _ _ _ _ _ w451 _ _ _ _ _ _ _ _]
          seq-local: [_ _ _ _ w440 _ _ _ _ _ _ _ _ _ _] -> [_ _ _ _ _ _ w450 _ _ _ _ _ _ _ _]
          seq-local: [_ _ _ _ _ _ w458 _ _ _ _ _ _ _ _] -> [_ _ _ _ _ _ _ _ w469 _ _ _ _ _ _]
          seq-local: [_ _ _ _ _ _ w457 _ _ _ _ _ _ _ _] -> [_ _ _ _ _ _ _ _ w468 _ _ _ _ _ _]
          seq-local: [_ _ _ _ _ _ _ _ w462 _ _ _ _ _ _] -> [_ _ _ _ _ _ _ _ _ _ w475 _ _ _ _]
          seq-local: [_ _ _ _ _ _ _ _ w461 _ _ _ _ _ _] -> [_ _ _ _ _ _ _ _ _ _ _ _ _ _ _]
          seq-local: [_ _ _ _ _ _ _ _ _ _ w471 _ _ _ _] -> [_ _ _ _ _ _ _ _ _ _ _ _ w485 _ _]
          seq-local: [_ _ _ _ _ _ _ _ _ _ w472 _ _ _ _] -> [_ _ _ _ _ _ _ _ _ _ _ _ w484 _ _]
          seq-local: [_ _ _ _ _ _ _ _ _ _ _ _ w483 _ _] -> [_ _ _ _ _ _ _ _ _ _ _ _ _ _ w496]
          seq-local: [_ _ _ _ _ _ _ _ _ _ _ _ w482 _ _] -> [_ _ _ _ _ _ _ _ _ _ _ _ _ _ w495]
          tunnel: w415 -> [w426 _ _ _ _ _ _ _ _ _ _ _ _ _ _]
          tunnel: w416 -> [w419 _ _ _ _ _ _ _ _ _ _ _ _ _ _]
          tunnel: w412 -> [w418 _ w432 _ w439 _ w455 _ w466 _ w476 _ w486 _ w499]
          tunnel: [_ _ _ _ _ _ _ _ _ _ _ _ _ _ w494] -> w411
          tunnel: [_ _ _ _ _ _ _ _ _ _ _ _ _ _ w493] -> w410
          frame #0 {
            w423 = " PULSe"  # Function Command
            n196 = local read "输出信号波形"() -> (w417:u16)
            n197 = Concatenate Strings(w418, ":FUNC" ("string (\"\")")) -> (w424:string)
            n198 = Pick Line(string ("")=w424, multi-line string=w423, line index=w417) -> (output string=w422:string)
            n199 = VISA Write(VISA resource name=w426, write buffer=w422, error in (no error)=w419) -> (VISA resource name out=w421:refnum<visa-resource-name>, error out=w420:errorcluster)  [unwired: 1 out]
          }
          frame #1 {
            n200 = Wait (ms)(milliseconds to wait=u32 150) -> ()  [unwired: 1 out]
          }
          frame #2 {
            n201 = Number To Fractional String(use system decimal point (T)=TRUE ("使用系统小数点(T)"), number="低电平/V") -> (F-format string=w430:string)  [unwired: 2 in]
            n202 = Concatenate Strings ("连接字符串")(w432, ":VOLTage:LOW ", w430) -> (w429:string)
            n203 = VISA Write(VISA resource name=w436, write buffer=w429, error in (no error)=w435) -> (VISA resource name out=w434:refnum<visa-resource-name>, error out=w433:errorcluster)  [unwired: 1 out]
          }
          frame #3 {
            n204 = Wait (ms)(milliseconds to wait=u32 150) -> ()  [unwired: 1 out]
          }
          frame #4 {
            # "1 频率"
            n205 = Concatenate Strings(w439, ":FREQ ") -> (w446:string)
            n206 = Format Into String ("格式化写入字符串")(initial string=w446, "频率/Hz") -> (resulting string=w447:string)  [unwired: 2 in, 1 out]
            n207 = VISA Write(VISA resource name=w445, write buffer=w447, error in (no error)=w444) -> (VISA resource name out=w443:refnum<visa-resource-name>, error out=w440:errorcluster)  [unwired: 1 out]
          }
          frame #5 {
            n208 = Wait (ms)(milliseconds to wait=u32 150) -> ()  [unwired: 1 out]
          }
          frame #6 {
            n209 = Number To Fractional String(use system decimal point (T)=TRUE ("使用系统小数点(T)"), number="高电平/V") -> (F-format string=w452:string)  [unwired: 2 in]
            n210 = Concatenate Strings(w455, ":VOLTage:HIGH ", w452) -> (w454:string)
            n211 = VISA Write(VISA resource name=w451, write buffer=w454, error in (no error)=w450) -> (VISA resource name out=w458:refnum<visa-resource-name>, error out=w457:errorcluster)  [unwired: 1 out]
          }
          frame #7 {
            n212 = Wait (ms)(milliseconds to wait=u32 150) -> ()  [unwired: 1 out]
          }
          frame #8 {
            n213 = local read "channel输出口"() -> (w464:i32)
            n214 = Pick Line(multi-line string=":OUTP1:IMPedance \n:OUTP2:IMPedance " ("write buffer"), line index=w464) -> (output string=w463:string)  [unwired: 1 in]
            n215 = Concatenate Strings ("连接字符串")(w466, w463, "INFINITY") -> (w467:string)
            n216 = VISA Write(VISA resource name=w469, write buffer=w467, error in (no error)=w468) -> (VISA resource name out=w462:refnum<visa-resource-name>, error out=w461:errorcluster)  [unwired: 1 out]
          }
          frame #9 {
            n217 = Wait (ms)(milliseconds to wait=u32 150) -> ()  [unwired: 1 out]
          }
          frame #10 {
            n218 = Number To Fractional String(use system decimal point (T)=TRUE ("使用系统小数点(T)"), number="占空比/%") -> (F-format string=w478:string)  [unwired: 2 in]
            n219 = Concatenate Strings(w476, ":PULSe:DCYCle ", w478) -> (w473:string)
            n220 = VISA Write(VISA resource name=w475, write buffer=w473, error in (no error)=w474) -> (VISA resource name out=w471:refnum<visa-resource-name>, error out=w472:errorcluster)  [unwired: 1 out]
          }
          frame #11 {
            n221 = Wait (ms)(milliseconds to wait=u32 150) -> ()  [unwired: 1 out]
          }
          frame #12 {
            n222 = Number To Fractional String(use system decimal point (T)=TRUE ("使用系统小数点(T)"), number="延时/s") -> (F-format string=w489:string)  [unwired: 2 in]
            n223 = Concatenate Strings(w486, ":PULSe:DELay ", w489) -> (w487:string)
            n224 = VISA Write(VISA resource name=w485, write buffer=w487, error in (no error)=w484) -> (VISA resource name out=w483:refnum<visa-resource-name>, error out=w482:errorcluster)  [unwired: 1 out]
          }
          frame #13 {
            n225 = Wait (ms)(milliseconds to wait=u32 150) -> ()  [unwired: 1 out]
          }
          frame #14 {
            w500 = ":LEADing\n:TRAiling "  # Channel
            w505 = ":PULSe:TRANsition"  # VOLTage:Offset
            n226 = local read "上升下降沿"() -> (w501:i32)
            n227 = Pick Line(multi-line string=w500, line index=w501) -> (output string=w497:string)  [unwired: 1 in]
            n228 = Number To Fractional String(use system decimal point (T)=TRUE ("使用系统小数点(T)"), number="上升下降沿/s") -> (F-format string=w498:string)  [unwired: 2 in]
            n229 = Concatenate Strings(w499, w505, w497, w498) -> (w502:string)
            n230 = VISA Write(VISA resource name=w496, write buffer=w502, error in (no error)=w495) -> (VISA resource name out=w494:refnum<visa-resource-name>, error out=w493:errorcluster)  [unwired: 1 out]
          }
        }
        n231 = VISA Close(VISA resource name=w411, error in (no error)=w410) -> (error out=→"configure error out":errorcluster)
      }
    }
    n232 = event shown="[1] \"照明光\": 值改变" {
      selector: _ -> [_ _]
      dyn-events: _ -> [_ _]
      timeout: 0 -> [_ _]
      tunnel: "照明光" -> [_ w23]
      event Timeout {
        n233 = event-data() -> ()  [unwired: 1 in, 3 out]
      }
      event "照明光": Value Change {
        n234 = event-data() -> ()  [unwired: 1 in, 6 out]
        n235 = local read "stop bits (10: 1 bit)"() -> (w36:u16)
        n236 = local read "parity (0:none)"() -> (w35:enum16{"None", "Odd", "Even", "Mark", "Space"})
        n237 = local read "照明光VISA"() -> (w32:refnum<visa-resource-name>)
        n238 = local read "baud rate"() -> (w33:u32)
        n239 = local read "data bits (8)"() -> (w34:u16)
        n240 = call-poly "VISA Configure Serial Port"("VISA resource name"=w32, "baud rate (9600)"=w33, "data bits (8)"=w34, "parity (0:none)"=w35, "stop bits (10: 1 bit)"=w36) -> ("VISA resource name out"=w29:refnum<visa-resource-name>, "error out"=w28:errorcluster)  [unwired: 9 in]
        n241 = call <vilib>:"Simple Error Handler.vi"("error in (no error)"=w28) -> ()  [unwired: 4 in, 5 out]
        n242 = VISA Open(access mode=0, error in (no error)=w28, VISA resource name=w29) -> (VISA resource name=w31:refnum<visa-resource-name>, error out=w30:errorcluster)  [unwired: 2 in]
        n243 = stacked-sequence {
          tunnel: w31 -> [w41]
          tunnel: w30 -> [w40]
          tunnel: [w39] -> w26
          tunnel: [w38] -> w27
          tunnel: w23 -> [w37]
          frame #0 {
            n244 = case shown="假" w37 {
              tunnel: w41 -> [w47 w57]
              tunnel: [w45 w56] -> w39
              tunnel: w40 -> [w46 w55]
              tunnel: [w44 w54] -> w38
              frame False {
                n245 = Concatenate Strings(" \u0001\u0001¢", "\r") -> (w48:string)
                n246 = VISA Write(VISA resource name=w47, write buffer=w48, error in (no error)=w46) -> (VISA resource name out=w45:refnum<visa-resource-name>, error out=w44:errorcluster)  [unwired: 1 out]
                n247 = Wait (ms)(milliseconds to wait=50) -> ()  [unwired: 1 out]
              }
              frame True {
                w50 = " \u0001\u0000¡"  # Channel
                n248 = Wait (ms)(milliseconds to wait=50) -> ()  [unwired: 1 out]
                n249 = Concatenate Strings(w50, "\r") -> (w51:string)
                n250 = VISA Write(VISA resource name=w57, write buffer=w51, error in (no error)=w55) -> (VISA resource name out=w56:refnum<visa-resource-name>, error out=w54:errorcluster)  [unwired: 1 out]
              }
            }
          }
        }
        n251 = VISA Close(VISA resource name=w26, error in (no error)=w27) -> (error out=w25:errorcluster)
        n252 = call <vilib>:"Simple Error Handler.vi"("error in (no error)"=w25) -> ()  [unwired: 4 in, 5 out]
      }
    }
  }
  n253 = flat-sequence {
    frame #0 {
      "Backlight" <- i32[][] [] ("Backlight")
    }
    frame #1 {
      w507 = FALSE
      # "删除背景光控件\n初始值设定"
      n254 = local write "cut backlight"(w507) -> ()
      "backlight" <- w507
    }
  }
  n255 = stacked-sequence {
    seq-local: [_ _ _ w528 _ _ _ _] -> [_ _ _ _ w546 w566 w569 w771]
    seq-local: [_ _ _ w527 _ _ _ _] -> [_ _ _ _ w547 w567 w568 w772]
    frame #0 {
      # "initialize all variables"
      n256 = property on="initialize" class="Bool"("Désactivé"=u8 0) -> ()  [unwired: 2 in, 2 out]
      n257 = property on="Acquire" class="Bool"("Visible"=FALSE) -> ()  [unwired: 2 in, 2 out]
      n258 = property on="Setup" class="Bool"("Visible"=FALSE) -> ()  [unwired: 2 in, 2 out]
      n259 = local write "indicator"("" ("indicator")) -> ()
      n260 = local write "initialized ?"(FALSE ("initialized ?")) -> ()
      n261 = local write "Continuous"(FALSE ("Continuous")) -> ()
      n262 = local write "Close"(FALSE ("Close")) -> ()
      n263 = property on="Device Name" class="Ring (严格)"("Désactivé"=u8 0) -> ()  [unwired: 2 in, 2 out]
      n264 = property on="Continuous" class="Bool (严格)"("Visible"=FALSE) -> ()  [unwired: 2 in, 2 out]
      n265 = local write "Commande tab"(T1."Settings" ("Commande tab")) -> ()
    }
    frame #1 {
      # "Read Uniq ID"
      n266 = stacked-sequence {
        frame #0 {
          n267 = call "read detector uniq-id.vi"() -> ("nbr of components"=w520:i32, "UniqueID"=w519:string[], "Name"=w518:string[])  [unwired: 4 out]
          n268 = for {
            N: w520 -> [_]
            tunnel: w519 -> [w522]
            tunnel: w518 -> [w521]
            n269 = property on="Device Name" class="Ring (严格)"("Chaînes []"=w521) -> ()  [unwired: 2 in, 2 out]
            n270 = property on="Uniques ID" class="Ring (严格)"("Chaînes []"=w522) -> ()  [unwired: 2 in, 2 out]
          }
        }
      }
    }
    frame #2 {
      n271 = while {
        stop <- "initialize" stop-if-true
        n272 = local read "Device Name"() -> (w525:u16)
        n273 = local write "Uniques ID"(w525) -> ()
        n274 = local read "Close"() -> (w523:bool)
        n275 = Stop(stop? (T)=w523) -> ()
        n276 = Wait Until Next ms Multiple(millisecond multiple=u32 100 ("n millisecondes")) -> ()  [unwired: 1 out]
      }
    }
    frame #3 {
      n277 = stacked-sequence {
        tunnel: [_ w535 _ _] -> w528
        tunnel: [_ w534 _ _] -> w527
        frame #0 {
          n278 = local write "indicator"("Initializing ..." ("indicator")) -> ()
        }
        frame #1 {
          n279 = local read "Uniques ID"() -> (w532:u16)
          n280 = property on="Uniques ID" class="Ring (严格)"() -> ("Chaînes []"=w533:string[])  [unwired: 2 in, 2 out]
          n281 = Index Array(array=w533, index=w532) -> (element=w531:string)
          n282 = call "Initialize CCD.vi"("Unique id:"=w531) -> ("activeYPixels"=→"Y Pixels:":i32, "JYCCDLib.IJYCCDReqd"=w534:refnum<k7>, "activeXPixels"=→"X Pixels:":i32, "sortie d'erreur"=w535:errorcluster, "FirmwareVersion"=→"Firmware\nVersion":string)  [unwired: 3 out]
        }
        frame #2 {
          n283 = property on="initialize" class="Bool"("Désactivé"=u8 2) -> ()  [unwired: 2 in, 2 out]
          n284 = property on="Device Name" class="Ring (严格)"("Désactivé"=u8 2) -> ()  [unwired: 2 in, 2 out]
          n285 = local write "Continuous"(FALSE ("Continuous")) -> ()
          n286 = property on="Setup" class="Bool"("Visible"=TRUE) -> ()  [unwired: 2 in, 2 out]
        }
        frame #3 {
          n287 = local write "initialized ?"(TRUE ("initialized ?")) -> ()
          n288 = local write "indicator"("Initialized !" ("indicator")) -> ()
        }
      }
    }
    frame #4 {
      # "Actually not working"
      # "Read ADC and GAIN"
      n289 = case shown="真" "Constante de condition\n(Voir l'aide contextuelle)" {
        tunnel: w547 -> [_ w557]
        tunnel: w546 -> [_ w556]
        frame False {
        }
        frame True {
          # "Read Input supported trigger"
          n290 = call "Trigger - Get Supported Input.vi"("JYCCDLib.IJYCCDReqd"=w557, "Error Input"=w556) -> ("trigAddress"=w551:i32, "eventPtr"=w552:i32, "trigEventString"=w555:string, "trigSigType"=w554:i32, "trigSigTypeString"=w553:string)  [unwired: 4 out]
          n291 = local write "trigSigTypeString"(w553) -> ()
          n292 = local write "trigAddress"(w551) -> ()
          n293 = local write "Trigger Type :"(w552) -> ()
          n294 = local write "trigEventString"(w555) -> ()
          n295 = local write "Signal type :"(w554) -> ()
        }
      }
      n296 = call "Init ADC & Gain.vi"("JYCCDLib.IJYCCDReqd"=w547, "input error"=w546) -> ("ADC Number"=w545:i32[], "ADC description"=w550:string[], "Gain Number"=w548:i32[], "Gain description"=w549:string[])
      n297 = local write "Gain Number"(w548) -> ()
      n298 = local write "ADC Number"(w545) -> ()
      n299 = stacked-sequence {
        tunnel: w550 -> [w558 _]
        tunnel: w549 -> [_ w559]
        frame #0 {
          n300 = property on="ADC" class="Ring (严格)"("Chaînes []"=w558) -> ()  [unwired: 2 in, 2 out]
        }
        frame #1 {
          n301 = property on="GAIN" class="Ring (严格)"("Chaînes []"=w559) -> ()  [unwired: 2 in, 2 out]
        }
      }
    }
    frame #5 {
      # "IS multi Accumulation Supported ?"
      n302 = call "MultiAccu - Is Supported.vi"("Error In"=w566, "JYCCDLib.IJYCCDReqd"=w567) -> ("IsOperatingModeSupported"=w560:bool)  [unwired: 3 out]
      n303 = Select(t=0, s=w560, f=2) -> (s? t:f=w563:i32)
      n304 = Select(t=FALSE, s=w560, f=w560) -> (s? t:f=w562:bool)
      n305 = local write "Multi Accumulation mode:"(w562) -> ()
      n306 = property on="Multi Accumulation mode:" class="Bool (严格)"("Désactivé"=w563) -> ()  [unwired: 2 in, 2 out]
      n307 = property on="Multi Accumulation mode:" class="Bool (严格)"("Désactivé"=w563) -> ()  [unwired: 2 in, 2 out]
    }
    frame #6 {
      n308 = while {
        tunnel: w568 -> [w576]
        tunnel: w569 -> [w575]
        stop <- "Close" stop-if-true
        n309 = local read "Continuous"() -> (w577:bool)
        n310 = case shown="假" "Reformat" {
          frame False {
          }
          frame True {
            n311 = local read "Y Pixels:"() -> (w749:i32)
            n312 = local read "X Pixels:"() -> (w751:i32)
            n313 = call "Spectral Reformat CCD area.vi"("Y Pixels:"=w749, "X Pixels:"=w751, "numAreas"="Number of Areas :") -> ("areas :"=→"areas :":i32[][])  [unwired: 3 out]
          }
        }
        n314 = local read "Accumulations:"() -> (w572:u16)
        n315 = Or(x="Acquire", y=w577) -> (x .or. y?=w574:bool)
        n316 = case shown="真" w574 {
          tunnel: w576 -> [_ w589]
          tunnel: w575 -> [_ w588]
          tunnel: "Enable InputTriggers :" -> [_ w587]
          tunnel: "Multi Accumulation mode:" -> [_ w586]
          tunnel: w572 -> [_ w585]
          tunnel: "MultiAcqShutterMode" -> [_ w584]
          frame False {
          }
          frame True {
            n317 = stacked-sequence {
              seq-local: [_ _ w602 _ _] -> [_ _ _ w675 _]
              seq-local: [_ _ _ w648 _] -> [_ _ _ _ w715]
              tunnel: w589 -> [_ w591 w606 w674 _]
              tunnel: w588 -> [_ w592 w605 w673 _]
              tunnel: w587 -> [_ w593 _ _ _]
              tunnel: w586 -> [_ _ w604 _ _]
              tunnel: w585 -> [_ _ w603 _ _]
              tunnel: w584 -> [_ _ w601 _ _]
              frame #0 {
                n318 = local write "CCD Busy"(TRUE ("CCD Busy")) -> ()
              }
              frame #1 {
                n319 = case shown="真" w593 {
                  tunnel: w592 -> [w594 w600]
                  tunnel: w591 -> [w595 w599]
                  frame False {
                    n320 = call "Trigger - Disable.vi"("Error In"=w594, "JYCCDLib.IJYCCDReqd"=w595) -> ()  [unwired: 6 out]
                  }
                  frame True {
                    n321 = local read "Trigger Type :"() -> (w596:u16)
                    n322 = local read "Signal type :"() -> (w597:enum16{"TTL Rising Edge", "TTL Falling Edge"})
                    n323 = local read "trigAddress"() -> (w598:i32)
                    n324 = call "Trigger - Enable.vi"("Error In"=w600, "sigType"=w597, "event"=w596, "trigAddress"=w598, "JYCCDLib.IJYCCDReqd"=w599) -> ()  [unwired: 3 out]
                  }
                }
              }
              frame #2 {
                n325 = case shown="真" w604 {
                  selector: w604 -> [_ w635]
                  tunnel: w606 -> [w632 w638]
                  tunnel: w605 -> [w631 w637]
                  tunnel: w603 -> [_ w636]
                  tunnel: [u16 1 ("Accumulations:") w636] -> w602
                  tunnel: w601 -> [_ w634]
                  frame False {
                    n326 = call "MultiAccu - Disable.vi"("Error In"=w631, "JYCCDLib.IJYCCDReqd"=w632) -> ()  [unwired: 4 out]
                  }
                  frame True {
                    n327 = call "MultiAccu - Configure.vi"("JYCCDLib.IJYCCDReqd"=w638, "Cleans Before"="Number of Cleans", "Accumulations:"=w636, "MultiAcqHardwareMode"=w635, "MultiAcqShutterMode"=w634, "Error In"=w637) -> ()  [unwired: 1 in, 9 out]
                  }
                }
                n328 = flat-sequence {
                  frame #0 {
                    n329 = Current VI's Path() -> (path=w612:path)
                    n330 = Get Date/Time In Seconds() -> (seconds since 1Jan1904=w614:timestamp)
                    n331 = Strip Path(path=w612) -> (stripped path=w613:path)  [unwired: 1 out]
                    n332 = Path To String(path=w613) -> (string=w615:string)
                    n333 = Format Date/Time String(time format string (%c)="%m.%d" ("时间格式字符串(%c)"), seconds (now)=w614) -> (date/time string=w621:string)  [unwired: 1 in]
                    n334 = Concatenate Strings(w615, "\\Save\\" ("字符串"), w621) -> (w616:string)
                    n335 = String To Path(string=w616) -> (path=w617:path)
                    n336 = call <vilib>:"Check if File or Folder Exists.vi"("path"=w617) -> ("file or folder exists?"=w618:bool, "dup path"=w620:path)  [unwired: 8 in, 1 out]
                    n337 = case shown="真" w618 {
                      tunnel: [w628 w629] -> w619
                      tunnel: w620 -> [w627 w629]
                      tunnel: w621 -> [w626 _]
                      frame False {
                        n338 = Create Folder(prompt (Create Folder)=w626, path (use dialog)=w627) -> (created path=w628:path)  [unwired: 1 in, 2 out]
                      }
                      frame True {
                      }
                    }
                    n339 = Format Date/Time String(time format string (%c)="%y%m%d%H%M%S " ("时间格式字符串(%c)"), seconds (now)=w614) -> (date/time string=w624:string)  [unwired: 1 in]
                    n340 = Path To String(path=w619) -> (string=w622:string)
                    n341 = Concatenate Strings(w622, "\\" ("字符串")) -> (w623:string)
                    n342 = Concatenate Strings(w623, w624) -> (w611:string)
                    n343 = String To Path(string=w611) -> (path=→"最终存储路径 2":path)
                  }
                }
              }
              frame #3 {
                n344 = local read "cut backlight"() -> (w662:bool)
                n345 = local read "backlight"() -> (w661:bool)
                n346 = call "MultiAccu - Acquire spectral.vi"("error in"=w673, "Accumulations:"=w675, "ShutterOpen"="ShutterOpen", "JYCCDLib.IJYCCDReqd"=w674) -> ("Acq Time(ms)"=→"Acq Time(ms)":u32, "Array Out"=w672:i32[][][])  [unwired: 1 out]
                n347 = And(x=w662, y=w661) -> (x .and. y?=w663:bool)
                n348 = call "Array reset dimension.vi"("Area Number"="Area Number to Display", "Array In"=w672) -> ("Array Out"=w664:i32[][])
                n349 = case shown="真" w663 {
                  tunnel: [w711 w712] -> w665
                  tunnel: w664 -> [w711 w713]
                  frame False {
                  }
                  frame True {
                    n350 = local read "Backlight"() -> (w714:i32[][])
                    n351 = Subtract(x=w713, y=w714) -> (x-y=w712:i32[][])
                  }
                }
                n352 = local read "波长范围"() -> (w640:dbl[])
                n353 = local write "Data"(w664) -> ()
                n354 = Index Array(array=w665, index (row)=0 ("禁用的索引 (列)")) -> (element=w666:i32[])  [unwired: 1 in]
                n355 = Reverse 1D Array(array=w666) -> (reversed array=w649:i32[])
                n356 = call "转换至动态数据2"("Array"=w640) -> ("Dynamic Data Type"=w668:dynamicdata)  [unwired: 3 in]
                n357 = call "转换至动态数据"("Array"=w649) -> ("Dynamic Data Type"=w669:dynamicdata)  [unwired: 3 in]
                n358 = call <vilib>:"Median Filter.vi"("left rank"=6, "X"=w649) -> ("Filtered X"=w654:dbl[])  [unwired: 8 in, 1 out]
                n359 = call "Build XY Graph2"("Y Input"=w669, "X Input"=w668) -> ("XY Graph"=w667:cluster{"Y":dbl[], "Y":dbl[]}[])  [unwired: 8 in, 1 out]
                n360 = Subtract(x="拟合终点", y="拟合起点") -> (x-y=w643:i32)
                n361 = local write "Spectrum"(w667) -> ()
                n362 = local read "滤波阈值"() -> (w658:dbl)
                n363 = Array Subset(array=w640, index="拟合起点", length=w643) -> (w646:dbl[])
                n364 = local read "拟合参数"() -> (w639:dbl[])
                n365 = In Range and Coerce(upper limit=w658, x=w654, lower limit=-100.0) -> (In Range?=w657:bool[])  [unwired: 1 out]
                n366 = Not(x=w657) -> (.not. x?=w651:bool[])
                n367 = local read "滤波阈值"() -> (w653:dbl)
                n368 = local write "范围内？"(w657) -> ()
                n369 = local read "X Pixels:"() -> (w655:i32)
                n370 = Or Array Elements(Boolean array=w651) -> (logical OR=w656:bool)
                n371 = case shown="真" w656 {
                  tunnel: w655 -> [_ w698]
                  tunnel: w654 -> [w694 w697]
                  tunnel: [w694 w696] -> w642
                  tunnel: w653 -> [_ w695]
                  frame False {
                  }
                  frame True {
                    n372 = for {
                      N: w698 -> [_]
                      tunnel: w697 -> [w702] mode=indexing
                      tunnel: [w701] -> w696 mode=indexing
                      shift-right: [w701] -> _
                      shift-left: _ -> [w700]
                      tunnel: w695 -> [w699]
                      n373 = Greater?(x=w702, y=w699) -> (0:w704:bool)
                      n374 = Less?(x=w702, y=-100.0) -> (x < y?=w705:bool)
                      n375 = Or(x=w704, y=w705) -> (x .or. y?=w703:bool)
                      n376 = case shown="真" w703 {
                        tunnel: w702 -> [w707 _]
                        tunnel: [w707 w709] -> w701
                        tunnel: w700 -> [_ w710]
                        frame False {
                        }
                        frame True {
                          n377 = call <vilib>:"Median Filter PtByPt.vi"("rank"=5, "x"=w710) -> ("Filtered x"=w709:dbl)  [unwired: 2 in, 1 out]
                        }
                      }
                    }
                  }
                }
                n378 = Array Subset(array=w642, index="拟合起点", length=w643) -> (w645:dbl[])
                n379 = Bundle("波长范围"=w640, "Filtered X"=w642) -> (w641:cluster{"波长范围 ":dbl[], "Filtered X":dbl[]})  [unwired: 1 in]
                n380 = case shown="真" "是否拟合" {
                  tunnel: w645 -> [w678 w684]
                  tunnel: w646 -> [_ w683]
                  tunnel: [w678 w682] -> w660
                  tunnel: w641 -> [_ w680]
                  frame False {
                  }
                  frame True {
                    n381 = call "转换至动态数据7"("Array"=w684) -> ("Dynamic Data Type"=w689:dynamicdata)  [unwired: 3 in]
                    n382 = call "转换至动态数据8"("Array"=w683) -> ("Dynamic Data Type"=w690:dynamicdata)  [unwired: 3 in]
                    n383 = call "曲线拟合2"("Locations"=w690, "Signals"=w689) -> ("best fit"=w687:dynamicdata, "non-linear coefficients"=w688:dynamicdata)  [unwired: 5 in, 3 out]
                    n384 = call "从动态数据转换3"("Dynamic Data Type"=w688) -> ("Array"=w691:dbl[])  [unwired: 3 in]
                    n385 = call "从动态数据转换4"("Dynamic Data Type"=w687) -> ("Array"=w682:dbl[])  [unwired: 3 in]
                    n386 = Index Array(array=w691, index #1=0 ("索引"), index #2=1 ("索引")) -> (element #1=w693:dbl, element #2=w692:dbl)
                    n387 = local write "拟合参数"(w691) -> ()
                    n388 = local write "xc"(w693) -> ()
                    n389 = Bundle(w683, "Array"=w682) -> (w681:cluster{dbl[], "Array":dbl[]})  [unwired: 1 in]
                    n390 = local write "w"(w692) -> ()
                    n391 = Build Array(w680, w681) -> (→"best fit":cluster{"波长范围 ":dbl[], "Array":dbl[]}[])
                  }
                }
                n392 = Build Array(w646, w649, w660, w639) -> (w648:dbl[][])
              }
              frame #4 {
                n393 = case shown="真" "是否保存" {
                  tunnel: w715 -> [_ w719]
                  frame False {
                  }
                  frame True {
                    n394 = Get Date/Time In Seconds() -> (seconds since 1Jan1904=w733:timestamp)
                    n395 = Get Date/Time String(date format (0)=enum16{"short", "long", "abbreviated"}."abbreviated" ("日期格式(0)"), seconds (now)=w733, want seconds? (F)=TRUE ("需要秒？(F)")) -> (date string=w731:string, time string=w732:string)
                    n396 = Search and Replace String(replace all?=TRUE ("替换全部？(F)"), input string=w732, search string=":" ("搜索字符串"), replace string="-" ("替换字符串(\"\")")) -> (result string=w730:string)  [unwired: 4 in, 3 out]
                    n397 = local read "最终存储路径 2"() -> (w734:path)
                    n398 = Path To String(path=w734) -> (string=w737:string)
                    n399 = Concatenate Strings(w737, w731, w730, "光谱" ("字符串"), ".xls" ("字符串")) -> (w736:string)
                    n400 = String To Path(string=w736) -> (path=w735:path)
                    n401 = call-poly <vilib>:"Write Delimited Spreadsheet.vi"("file path (dialog if empty)"=w735, "format (%.3f)"="%.16f", "2D data"=w719, "append to file? (new file:F)"=TRUE ("append to file? (F)"), "transpose? (no:F)"=TRUE ("transpose? (F)")) -> ()  [unwired: 9 in, 2 out]
                  }
                }
                n402 = case shown="真" "Save Backlight" {
                  frame False {
                  }
                  frame True {
                    w738 = TRUE ("删除背景光")
                    n403 = local read "Data"() -> (w740:i32[][])
                    n404 = local write "Backlight"(w740) -> ()
                    n405 = local write "cut backlight"(w738) -> ()
                    n406 = local write "backlight"(w738) -> ()
                    n407 = local write "Save Backlight"(FALSE ("Save Backlight")) -> ()
                  }
                }
                n408 = local write "CCD Busy"(FALSE ("CCD Busy")) -> ()
              }
            }
          }
        }
        n409 = case shown="假" "Setup" {
          tunnel: w575 -> [_ w754]
          tunnel: w576 -> [_ w753]
          frame False {
          }
          frame True {
            n410 = stacked-sequence {
              tunnel: w754 -> [_ w768 _]
              tunnel: w753 -> [_ w756 _]
              frame #0 {
                n411 = local write "indicator"("Setting up the detector" ("indicator")) -> ()
              }
              frame #1 {
                w766 = 1 items=["JYMCD_ACQ_FORMAT_IMAGE", "JYMCD_ACQ_FORMAT_SCAN"] ("Acquisition type")
                n412 = local read "Gain Number"() -> (w761:i32[])
                n413 = local read "GAIN"() -> (w757:u16)
                n414 = local read "ADC Number"() -> (w762:i32[])
                n415 = local read "ADC"() -> (w758:u16)
                n416 = Index Array(array=w761, index=w757) -> (element=w759:i32)
                n417 = Index Array(array=w762, index=w758) -> (element=w760:i32)
                n418 = local read "Number of Areas :"() -> (w764:u16)
                n419 = local read "areas :"() -> (w765:i32[][])
                n420 = call "Setup CCD.vi"("numAreas"=w764, "areas :"=w765, "JYCCDLib.IJYCCDReqd"=w756, "entrée d'erreur (pas d'erreur)"=w768, "Acquisition type"=w766, "Gain"=w759, "Select ADC"=w760, "Integration time(ms)"="Integration time (ms) :") -> ("DataSize"=→"DataSize":i32)  [unwired: 1 out]
                "JYCCDLib.IJYCCDReqd" <- w756
              }
              frame #2 {
                w769 = TRUE ("Visible")
                n421 = property on="Continuous" class="Bool (严格)"("Visible"=w769) -> ()  [unwired: 2 in, 2 out]
                n422 = property on="Acquire" class="Bool"("Visible"=w769) -> ()  [unwired: 2 in, 2 out]
                n423 = local write "indicator"("Ready !" ("indicator")) -> ()
              }
            }
          }
        }
        n424 = case shown="假" "Temperature" {
          tunnel: w576 -> [_ w743]
          tunnel: w575 -> [_ w742]
          frame False {
            n425 = property on="temp graph" class="WFChart (严格)"("Visible"=FALSE) -> ()  [unwired: 2 in, 2 out]
          }
          frame True {
            n426 = stacked-sequence {
              tunnel: w743 -> [_ w748]
              tunnel: w742 -> [_ w747]
              frame #0 {
                n427 = property on="temp graph" class="WFChart (严格)"("Visible"=TRUE) -> ()  [unwired: 2 in, 2 out]
              }
              frame #1 {
                w746 = u16 0 items=["° Celsius", "Kelvin", "° Farenheit"] ("units")
                n428 = call "read temperature.vi"("entrée d'erreur (pas d'erreur)"=w747, "units"=w746, "JYCCDLib.IJYCCDReqd"=w748) -> ("Current Temperature"=w745:dbl)
                n429 = local write "temp graph"(w745) -> ()
              }
            }
          }
        }
        n430 = Wait Until Next ms Multiple(millisecond multiple=u32 50 ("n millisecondes")) -> ()  [unwired: 1 out]
      }
    }
    frame #7 {
      n431 = Close Reference(reference=w772, error in (no error)=w771) -> ()  [unwired: 1 out]
    }
  }
  n432 = stacked-sequence {
    seq-local: [_ _ w782 _ _] -> [_ _ _ w792 w797]
    seq-local: [_ _ w781 _ _] -> [_ _ _ w791 _]
    seq-local: [_ _ _ w790 _] -> [_ _ _ _ _]
    frame #0 {
      n433 = call "Get Monos From Config Browser.vi"() -> ("UniqueIDs"=w777:string[], "Mono ID"=w778:string[])  [unwired: 3 in, 1 out]
      n434 = Build Cluster Array(w778, w777) -> (w775:cluster{"String":string, "String":string}[])
      n435 = property on="Mono ID" class="CmbBox"("Strings And Values []"=w775) -> ()  [unwired: 2 in, 2 out]
      n436 = Index Array(array=w775, index=0) -> (element=w776:cluster{"String":string, "String":string})
      n437 = Unbundle(w776) -> ("String"=w773:string)  [unwired: 1 out]
      "Current UniqueID" <- w773
      n438 = local write "Mono ID"(w773) -> ()
    }
    frame #1 {
      n439 = while {
        stop <- "Connect" stop-if-true
        n440 = local read "Mono ID"() -> (w779:string)
        n441 = local write "Current UniqueID"(w779) -> ()
      }
    }
    frame #2 {
      n442 = local read "Mono ID"() -> (w784:string)
      n443 = call "JYInitMono.vi"("Unique ID"=w784, "Force Init"="Force\nInitialization") -> ("Refnum out"=w782:refnum<k7>, "Initialized"=→"Initialized JY":bool, "error out"=w781:errorcluster)  [unwired: 9 in, 2 out]
    }
    frame #3 {
      n444 = call "Show Current Grating.vi"("Refnum in"=w792, "error in (no error)"=w791) -> ("Gratings"=w793:dbl[], "Grating Index"=w787:i32, "Current Grating"=w789:dbl, "Current Description"=w786:string, "error out"=w790:errorcluster)  [unwired: 5 in, 4 out]
      "Gratings" <- w793
      n445 = local write "Current Grating"(w789) -> ()
      n446 = local write "Current Description"(w786) -> ()
      n447 = Number To Decimal String(number=w793) -> (decimal integer string=w795:string[])  [unwired: 1 in]
      n448 = Number To Decimal String(number=w787) -> (decimal integer string=w788:string)  [unwired: 1 in]
      n449 = property on="Target Grating" class="CmbBox"("Value"=w788) -> ()  [unwired: 2 in, 2 out]
      n450 = Build Cluster Array(w795, string[] ["1", "2", "3"]) -> (w796:cluster{"Numeric":string, string}[])
      n451 = property on="Target Grating" class="CmbBox"("Strings And Values []"=w796) -> ()  [unwired: 2 in, 2 out]
    }
    frame #4 {
      n452 = while {
        tunnel: w797 -> [w799]
        stop <- w798 stop-if-true
        n453 = stacked-sequence {
          seq-local: [w803 _ _ _ _] -> [_ w810 w821 _ w829]
          seq-local: [w802 _ _ _ _] -> [_ w809 w820 _ _]
          seq-local: [_ w808 _ _ _] -> [_ _ _ _ _]
          seq-local: [_ w807 _ _ _] -> [_ _ _ _ _]
          seq-local: [_ _ w813 _ _] -> [_ _ _ _ _]
          seq-local: [_ _ w812 _ _] -> [_ _ _ w823 _]
          tunnel: w799 -> [w801 _ _ w824 _]
          frame #0 {
            n454 = call "Show Current Grating.vi"("Refnum in"=w801) -> ("Grating Index"=→"Grating Index":i32, "Current Grating"=→"Current Grating":dbl, "Current Description"=→"Current Description":string, "error out"=w802:errorcluster, "JYMONOLib.IJYMonoReqd"=w803:refnum<k7>)  [unwired: 6 in, 4 out]
          }
          frame #1 {
            n455 = call "JYGetCurrentWL.vi"("error in (no error)"=w809, "JYMONOLib.IJYMonoReqd"=w810) -> ("error out"=w807:errorcluster, "Units"=→"Units":string, "Current WL"=→"Current WL":dbl, "JYMONOLib.IJYMonoReqd 2"=w808:refnum<k7>)  [unwired: 6 in]
          }
          frame #2 {
            w818 = u16 1 items=["Entrance", "Exit"] ("Mirror Number")
            w819 = u16 0 items=["Entrance", "Exit"] ("Mirror Number")
            n456 = call "JYGetMirrorPos.vi"("error in (no error)"=w820, "Mirror"=w819, "Refnum In"=w821) -> ("error out"=w816:errorcluster, "Current Mirror Position"=→"Entrance Mirror\nPosition":i32, "Refnum Out"=w817:refnum<k7>)  [unwired: 1 in]
            n457 = call "JYGetMirrorPos.vi"("error in (no error)"=w816, "Mirror"=w818, "Refnum In"=w817) -> ("error out"=w812:errorcluster, "Current Mirror Position"=→"Exit Mirror\nPosition":i32, "Refnum Out"=w813:refnum<k7>)  [unwired: 1 in]
          }
          frame #3 {
            w826 = u16 0 items=["Front Entrance", "Side Entrance", "Front Exit", "Side Exit", "First Intermediate", "Second Intermediate"] ("Slit")
            n458 = call "JYGetSlits.vi"("MonoRefNum IN"=w824, "Slit"=w826, "error in (no error)"=w823) -> ("Units"=→"Units 2":string, "Slit Width"=→"Front Entrance":dbl, "error out"=→"error out":errorcluster)  [unwired: 13 in, 1 out]
          }
          frame #4 {
            n459 = case shown="假" "Move To\nTarget Positions" {
              tunnel: w829 -> [_ w830]
              frame False {
              }
              frame True {
                n460 = stacked-sequence {
                  seq-local: [w832 _ _ _] -> [_ w838 _ _]
                  seq-local: [_ w836 _ _] -> [_ _ w853 _]
                  seq-local: [_ _ w840 _] -> [_ _ _ w859]
                  seq-local: [_ _ _ w856] -> [_ _ _ _]
                  tunnel: w830 -> [w834 w837 w851 w860]
                  frame #0 {
                    n461 = property on="Target Grating" class="CmbBox"() -> ("Value"=w831:string)  [unwired: 2 in, 2 out]
                    n462 = local read "error out"() -> (w833:errorcluster)
                    n463 = Decimal String To Number(string=w831) -> (number=w835:i32)  [unwired: 2 in, 1 out]
                    n464 = call "JYTurret.vi"("error in (no error)"=w833, "Grating Index"=w835, "JYMONOLib.IJYMonoReqd"=w834) -> ("error out"=w832:errorcluster)  [unwired: 2 out]
                  }
                  frame #1 {
                    # "Move Grating to Target Position"
                    n465 = call "JYMoveToWavelength.vi"("error in (no error)"=w838, "Target WL"="Target WL", "RefNum In"=w837) -> ("error out"=w836:errorcluster)  [unwired: 1 in, 2 out]
                  }
                  frame #2 {
                    w846 = u16 1 items=["Entrance", "Exit"] ("Mirror Number")
                    w845 = u16 0 items=["Entrance", "Exit"] ("Mirror Number")
                    w852 = u16 1 items=["Entrance", "Exit", "Front", "Side"] ("Mirror Number")
                    w855 = u16 0 items=["Entrance", "Exit", "Front", "Side"] ("Mirror Number")
                    # "Move Mirrors"
                    n466 = call "JYMirrorMove.vi"("error in (no error)"=w853, "Mirror Position"="Entrance Mirror", "Mirror Number"=w855, "RefNum In"=w851) -> ("error out"=w850:errorcluster)  [unwired: 6 in, 1 out]
                    n467 = call "JYMirrorMove.vi"("error in (no error)"=w850, "Mirror Position"="Exit Mirror", "Mirror Number"=w852, "RefNum In"=w851) -> ("error out"=w843:errorcluster, "MonoRefNum Out"=w844:refnum<k7>)  [unwired: 6 in]
                    n468 = call "JYGetMirrorPos.vi"("error in (no error)"=w843, "Mirror"=w845, "Refnum In"=w844) -> ("error out"=w848:errorcluster, "Current Mirror Position"=w842:i32, "Refnum Out"=w847:refnum<k7>)  [unwired: 1 in]
                    n469 = local write "Entrance Mirror\nPosition"(w842) -> ()
                    n470 = call "JYGetMirrorPos.vi"("error in (no error)"=w848, "Mirror"=w846, "Refnum In"=w847) -> ("error out"=w840:errorcluster, "Current Mirror Position"=w841:i32)  [unwired: 1 in, 1 out]
                    n471 = local write "Exit Mirror\nPosition"(w841) -> ()
                  }
                  frame #3 {
                    w858 = u16 0 items=["Front Entrance", "Side Entrance", "Front Exit", "Side Exit", "First Intermediate", "Second Intermediate"] ("Slit")
                    # "Set New Slit Positions"
                    n472 = call "JYSlits.vi"("JYMONOLib.IJYMonoReqd"=w860, "Slit"=w858, "error in (no error)"=w859, "Slit Width"="Target\nFront Entrance") -> ("error out"=w856:errorcluster)  [unwired: 1 in, 1 out]
                  }
                }
              }
            }
          }
        }
        n473 = local read "Close"() -> (w798:bool)
      }
    }
  }
  n474 = flat-sequence {
    frame #0 {
      n475 = call <vilib>:"Create Report.vi"("window state (normal)"=T3."no change", "report type"=Report_Type."Excel", "template (empty)"=path "D:/desktop/train/TEST1/Save/2670中心波长.xlsx") -> ("report out"=w867:refnum<class "NI_report.lvclass">, "error out"=w866:errorcluster)  [unwired: 11 in]
      n476 = call-poly <vilib>:"Excel Get Data.vi"("report in"=w867, "data type"=string[][] [], "error in (no error)"=w866) -> ("report out"=w862:refnum<class "NI_report.lvclass">, "data"=w870:string[][], "error out"=w861:errorcluster)  [unwired: 10 in]
      n477 = call-dynamic "Dispose Report.vi"("report in"=w862, "error in (no error)"=w861) -> ()  [unwired: 13 in, 1 out]
      n478 = Index Array(array=w870, index (col)=0 ("禁用的索引 (列)")) -> (element=w872:string[])  [unwired: 1 in]
      n479 = Fract/Exp String To Number(string=w872) -> (number=→"波长范围":dbl[])  [unwired: 3 in, 1 out]
    }
  }
